vi "Simulation.Main.vi"() -> ()   [LabVIEW 2016, in "Simulation.lvclass"]
uses:
  Simulation.lvclass
  SimState.ctl
  Package ResourceControl/ViHandler/ViHandler.ViInfo.ctl
  SimModes.ctl
  Package Libraries/Message Queue/private/MessageQueue.MessageTypeDef.ctl
  <vilib>/Platform/TimedLoop/XDataNode/timing_clust.ctl
  <vilib>/Platform/TimedLoop/XDataNode/nitl_modes.ctl
  <vilib>/Platform/TimedLoop/XDataNode/wakeup.ctl
  Simulation.lvclass/Simulation.ctl
  Package ErrorHandling/ErrorHandling.lvclass/ErrorHandling.ctl
  Modell/Sondenmodell/Sondenmodell.lvclass/Sondenmodell.ctl
  Modell/Hausmodell/Hausmodell.lvclass/Hausmodell.ctl
  Modell/Umgebung/Umgebung.lvclass/Umgebung.ctl
  Package ErrorHandling/ErrorHandling.checkForErrorAndHandle.vi
  Package ErrorHandling/ErrorHandling.GetErrorHandler.vi
  <vilib>/Utility/error.llb/Clear Errors.vi
  Package Libraries/StringFunctions/StringFunctions_ReplaceAllBlindSigns.vi
  <vilib>/dlg_ctls.llb/Space Constant.vi
  <vilib>/Utility/error.llb/Error Cluster From Error Code.vi
  Package Libraries/TimingFunctions/TimingFunctions_getUtcTimestamp.vi
  <vilib>/Utility/error.llb/Trim Whitespace.vi
  <vilib>/Utility/error.llb/Search and Replace Pattern.vi
  Package ErrorHandling/ErrorHandling.addLastErrorToFile.vi
  <vilib>/ErrorRing/Error Ring.xnode
  Package ErrorHandling/ErrorHandling.lvclass
  <vilib>/Platform/TimedLoop/XDataNode/XDataNode.xnode
  <vilib>/Platform/TimedLoop/XDataNode/XDNodeRunTimeDep.lvlib
  Package ResourceControl/ViHandler/ViHandler.lvclass
  Modell/Sondenmodell/Sondenmodell.lvclass
  Modell/Umgebung/Umgebung.lvclass
  Modell/Hausmodell/Hausmodell.lvclass
panel:
  in  "Relative Zeit":timestamp=timestamp(3625116099.829659 s since 1904-01-01) format="%<%H:%M\n%d/%m/%Y>T"
  in  "Kalender und Uhrzeit Startwert":timestamp=timestamp(3625116099.829659 s since 1904-01-01) format="%<%H:%M\n%d/%m/%Y>T"
  in  "Umgebung":enum32{"Umgebung"}(tab)
  in  "Aussentemperatur [°C] Manuell":dbl(slide)=20.0 caption="Aussentemperatur [°C]" min=-20.0 max=40.0 scale=-20.0..40.0 scale format="%#.0f"
  in  "Manuelle Eingabe On/Off":bool
  out "Solare Gewinne [W]":dbl format="%#.0f"
  out "Strahlungsleistung  Sonne [W]":dbl format="%#.0f"
  in  "Kalender und Uhrzeit":timestamp=timestamp(3597606016.6082277 s since 1904-01-01) format="%<%H:%M\n%d/%m/%Y>T"
  out "Aussentemperatur":waveform(dbl)[](graph)
  in  "Solare Gewinne [W] Manuell":dbl(slide) caption="Solare Gewinne [W]" min=0.0 max=1000.0 scale=0.0..1000.0 scale format="%#.0f"
  in  "SimMode":T1
  in  "StopSim":bool
  in  "SimulationsModis":T2(tab)
  in  "Erdtemperatur [°C] Gesamtmodell":dbl=10.0 caption="Erdtemperatur [°C]" format="%#.0f"
  in  "Rücklauftemperatur Solekreislauf [°C] Gesamtmodell":dbl caption="Rücklauftemperatur Solekreislauf [°C]" format="%#.0f"
  in  "Rücklauftemperatur Heizkreislauf [°C] Gesamtmodell":dbl=25.0 caption="Rücklauftemperatur Heizkreislauf [°C]" format="%#.0f"
  in  "Bodentemperatur [°C] Gesamtmodell":dbl=20.0 caption="Bodentemperatur [°C]" format="%#.0f"
  in  "Raumtemperatur [°C] Gesamtmodell":dbl=15.0 caption="Raumtemperatur [°C]" format="%#.0f"
  in  "Verdichter 1 Gesamtmodell":bool caption="Verdichter 1"
  in  "Verdichter 2 Gesamtmodell":bool caption="Verdichter 2"
  out "Gesamtmodell":waveform(dbl)[](graph)
  out "Vorlauftemperatur Heizkreislauf [°C] Gesamtmodell":dbl=25.0 caption="Vorlauftemperatur Heizkreislauf [°C]" format="%#.0f"
  out "Vorlauftemperatur Solekreislauf [°C] Gesamtmodell":dbl caption="Vorlauftemperatur Solekreislauf [°C]" format="%#.0f"
  out "Hausmodell":waveform(dbl)[](graph)
  in  "Rücklauftemperatur Heizkreislauf [°C]":dbl=20.0 format="%#.0f"
  in  "Vorlauftemperatur \nHeizkreislauf [°C] Hausmodell":dbl(slide)=21.0 caption="Vorlauftemperatur \nHeizkreislauf [°C]" min=-20.0 max=60.0 scale=-20.0..60.0 scale format="%#_3p"
  in  "Bodentemperatur [°C]":dbl=18.0 format="%#.0f"
  in  "Raumtemperatur [°C]":dbl=16.0 format="%#.0f"
  in  "Erdtemperatur [°C]":dbl=10.0 min=0.0 max=20.0 format="%#.0f"
  in  "Rücklauftemperatur Solekreislauf [°C]":dbl=10.0 format="%#.0f"
  in  "Vorlauftemperatur \nSolekreislauf [°C] Sondemodell":dbl(slide)=9.0 caption="Vorlauftemperatur \nSolekreislauf [°C]" min=-10.0 max=20.0 scale=-10.0..20.0 scale format="%#.0f"
  out "Sondenmodell":waveform(dbl)[](graph)
  out "Vorlauftemperatur\n Solekreislauf [°C] Wärmepumpenmodell":dbl caption="Vorlauftemperatur\nSolekreislauf [°C]" format="%#.0f"
  out "Vorlauftemperatur\n Heizkreislauf [°C] Wärmepumpenmodell":dbl=35.0 caption="Vorlauftemperatur\nHeizkreislauf [°C]" format="%#.0f"
  out "Kälteleistung [W]":dbl format="%#.0f"
  out "Heizleistung [W]":dbl format="%#.0f"
  in  "Rücklauftemperatur \nSolekreislauf [°C] Wärmepumpenmodell":dbl(slide)=5.0 caption="Rücklauftemperatur \nSolekreislauf [°C]" min=-10.0 max=20.0 scale=-10.0..20.0 scale format="%#.0f"
  in  "Rücklauftemperatur Heizkreislauf  [°C] Wärmepumpenmodell":dbl(slide)=20.0 caption="Rücklauftemperatur \nHeizkreislauf [°C]" min=-20.0 max=60.0 scale=-20.0..60.0 scale format="%#.0f"
  in  "Verdichter 2 Wärmepumpenmodell":bool caption="Verdichter 2"
  in  "Verdichter 1 Wärmepumpenmodell":bool caption="Verdichter 1"
  out "ViInfo":T3
  in  "SetInitials":bool
  in  "PauseSim":bool
  in  "StartSim":bool
  in  "SimState":T4
  in  "Speed Multipier":i64=100
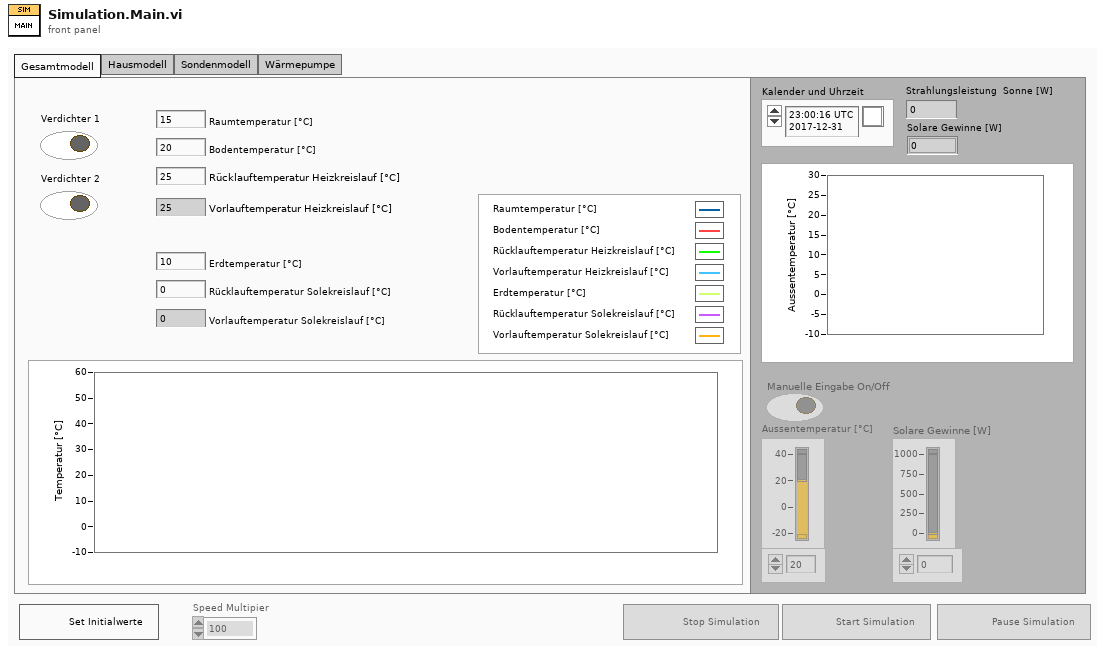
[diagram p1: front panel]
types:
  T1 = typedef "Simulation.lvclass/SimModes.ctl" = enum16{"Gesamtmodell", "HausOnly", "SondeOnly", "WPOnly"}
  T2 = enum32{"Gesamtmodell", "Hausmodell", "Sondenmodell", "Wärmepumpe"}
  T3 = typedef "ViHandler.lvclass/ViHandler.ViInfo.ctl" = cluster{"ViName":string, "ViReference":refnum<vi>, "ViQueueName":string}
  T4 = typedef "Simulation.lvclass/SimState.ctl" = enum16{"SetParams", "Running", "Idle", "Exit"}
  T5 = typedef "MessageQueue.MessageTypeDef.ctl" = cluster{"Message":string, "Data":variant}
  T6 = typedef "XDNodeRunTimeDep.lvlib/timing_clust.ctl" = cluster{"Expected End [f-1]":u64, "Actual End [f-1]":u64, "Finished Late? [f-1]":bool, "Expected End [i-1]":u64, "Actual End [i-1]":u64, "Finished Late? [i-1]":bool, "Expected Start [i]":u64, "Actual Start [i]":u64, "Expected Start [f]":u64, "Actual Start [f]":u64, "Source Name":string, "Structure Name":string, "Period":i64, "Deadline":i64, "Offset":i64, "Start":i64, "Priority":i32, "Timeout":i32, "Mode":T7, "Wakeup Reason":T8, "Error":errorcluster, "Source Type":string, "Secondary Source Type":string, "Global End Time":u64, "Global Start Time":u64, "Frame Duration":u64, "Iteration Duration":u64, "Assigned CPU":i32, "I/O Scan Engine Mode":u32}
  T7 = typedef "XDNodeRunTimeDep.lvlib/nitl_modes.ctl" = enum32{"No Change", "Process missed periods, maintain original phase", "Discard missed periods, maintain original phase", "Process missed periods, ignore original phase", "Discard missed periods, ignore original phase"}
  T8 = typedef "XDNodeRunTimeDep.lvlib/wakeup.ctl" = enum32{"Normal", "Aborted", "Asynchronous wakeup", "Timing source error", "Timed loop error", "Timeout"}
  T9 = enum8{"Enabled", "Disabled", "Disabled and Grayed Out"}
  T10 = enum32{"Page Enabled", "Page Disabled", "Page Disabled & Grayed"}
  T11 = typedef "Wärmepumpe.lvclass/Wärmepumpe.Zustandsgrössen.ctl" = cluster{"Vorlauftemperatur Heizkreislauf[°C]":dbl, "Vorlauftemperatur Solekreislauf[°C]":dbl, "Heizleistung [W]":dbl, "Kälteleistung [W]":dbl, "Verdichter 1":bool, "Verdichter 2":bool}
  T12 = typedef "Hausmodell.lvclass/Hausmodell.Zustandsgrössen.ctl" = cluster{"Raumtemperatur [°C]":dbl, "Bodentemperatur [°C]":dbl, "Rücklauftemperatur Heizkreislauf [°C]":dbl}
  T13 = typedef "Sondenmodell.lvclass/Sondenmodell.Zustandsgrössen.ctl" = cluster{"Erdtemperatur [°C]":dbl, "Rücklauftemperatur Solekreislauf [°C]":dbl}
  T14 = typedef "Umgebung.lvclass/Umgebung.Zustandsgrössen.ctl" = cluster{"Aussentemperatur [°C]":dbl, "Aussentemperatur [°C] Manuell":dbl, "Tag":dbl, "Stunde":dbl, "Minute":dbl, "Sekunden":dbl, "Strahlungsleistung [W]":dbl, "Solare Gewinne [W]":dbl, "Solare Gewinne [W] Manuell":dbl, "Manuelle Eingabe On/Off":bool}
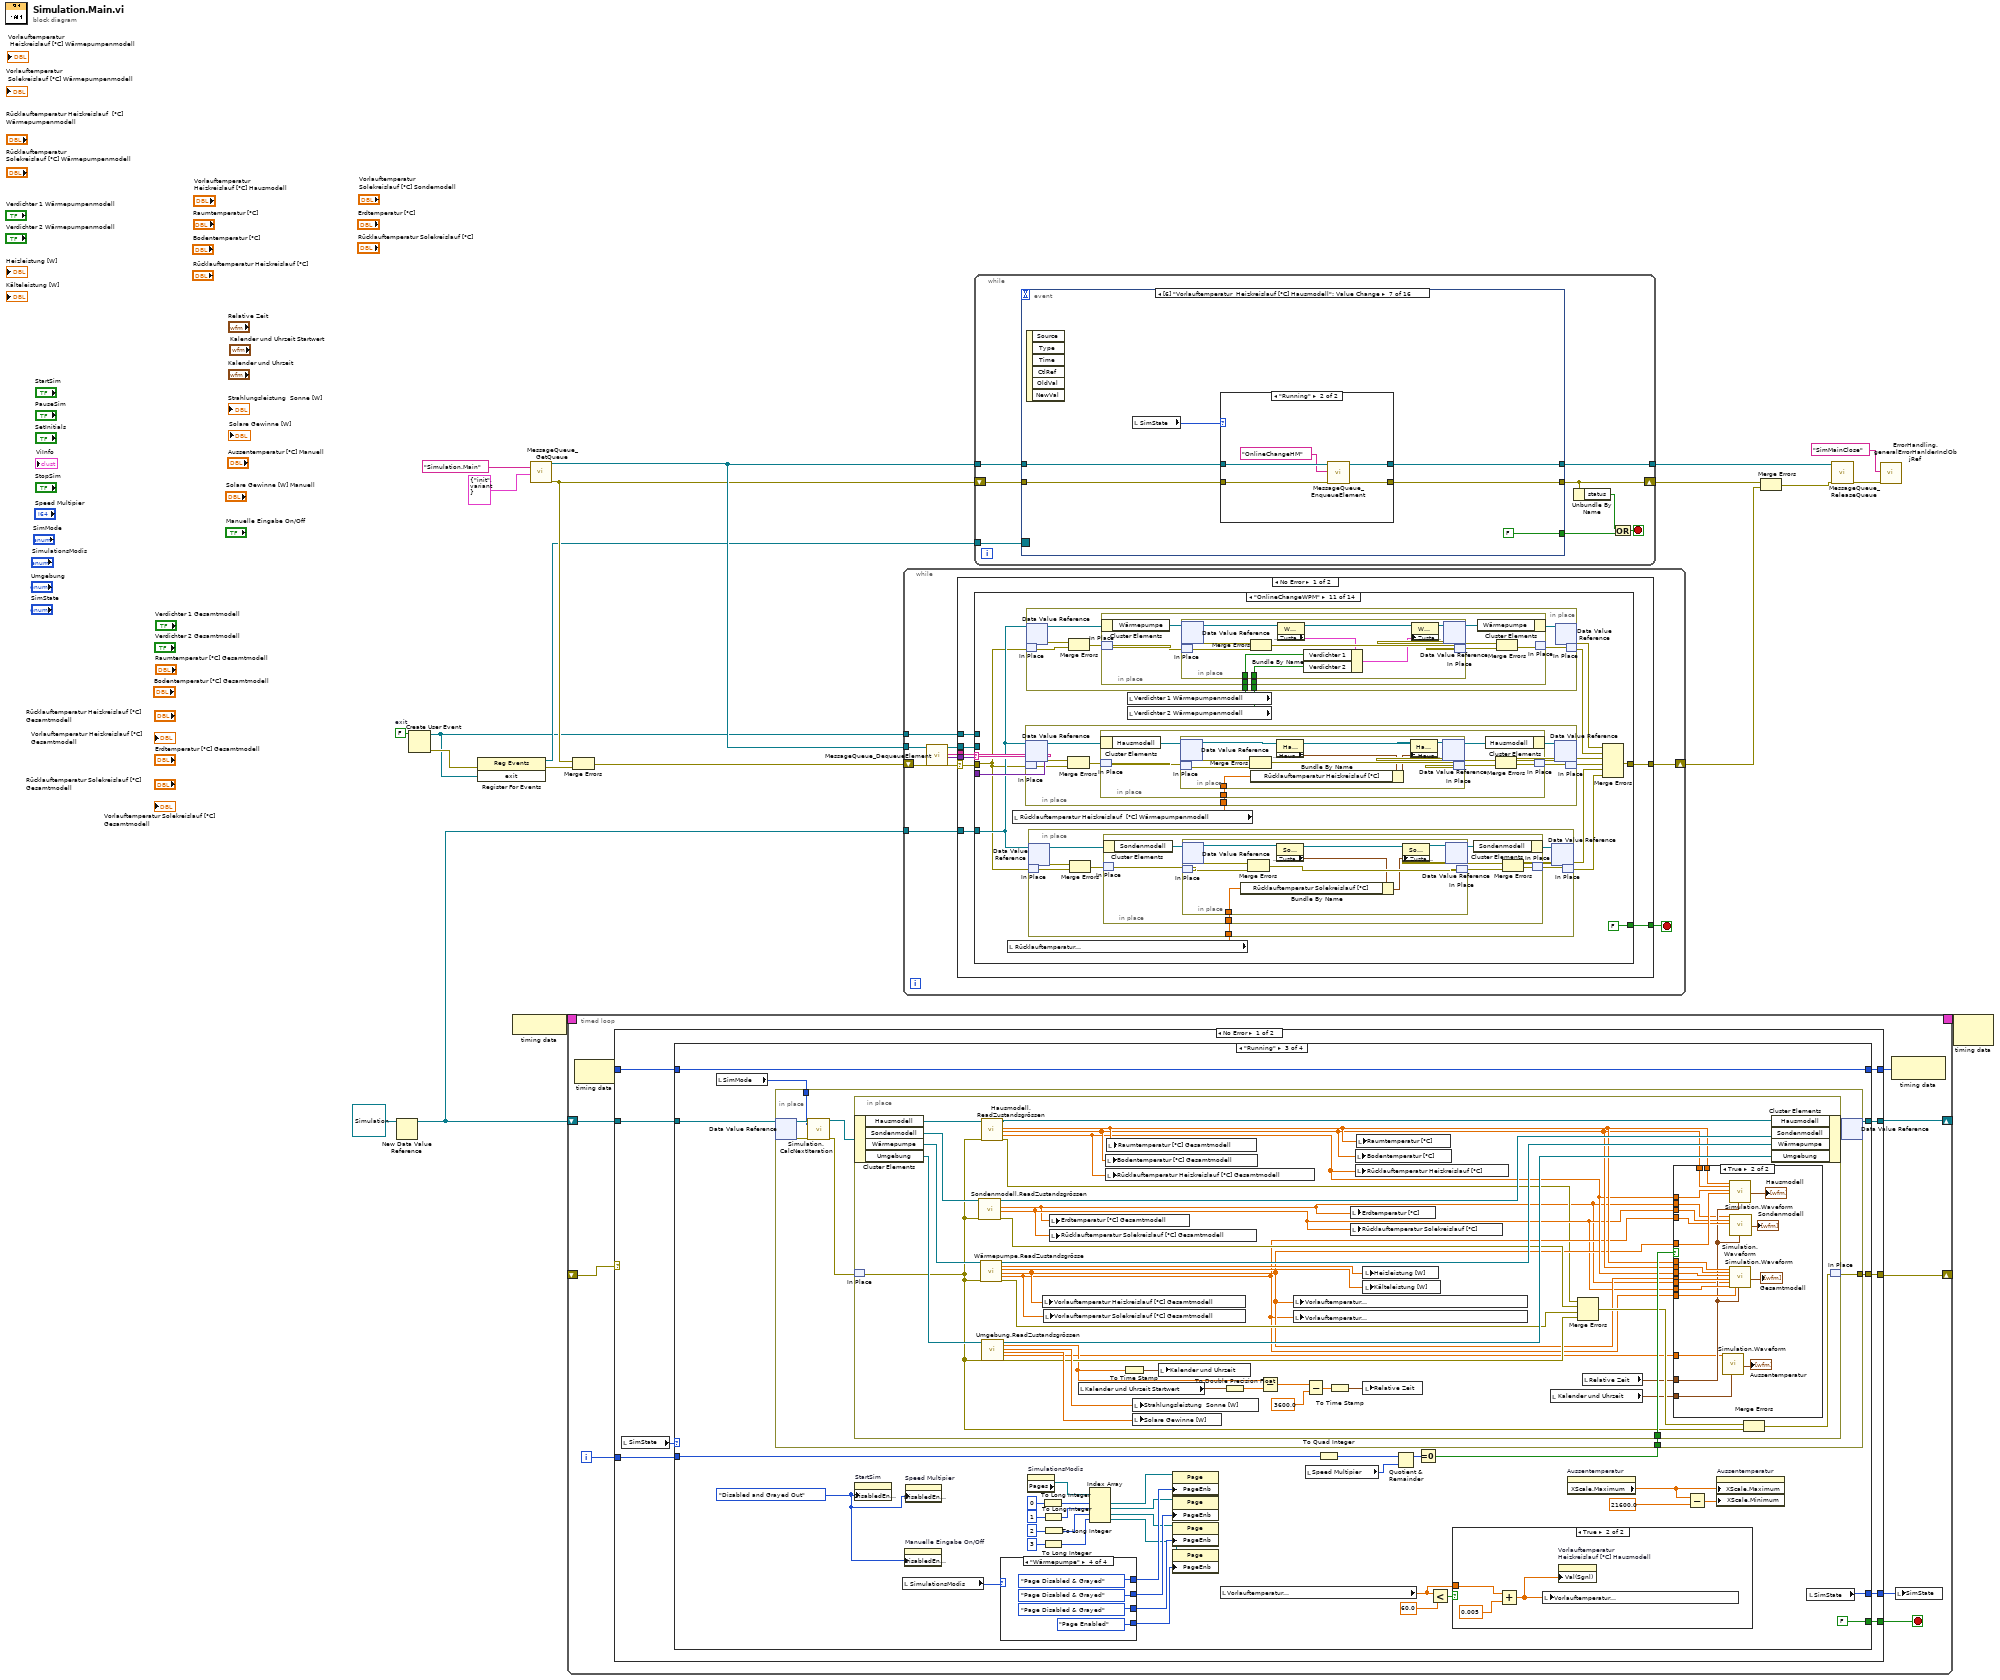
[diagram p0: block diagram]
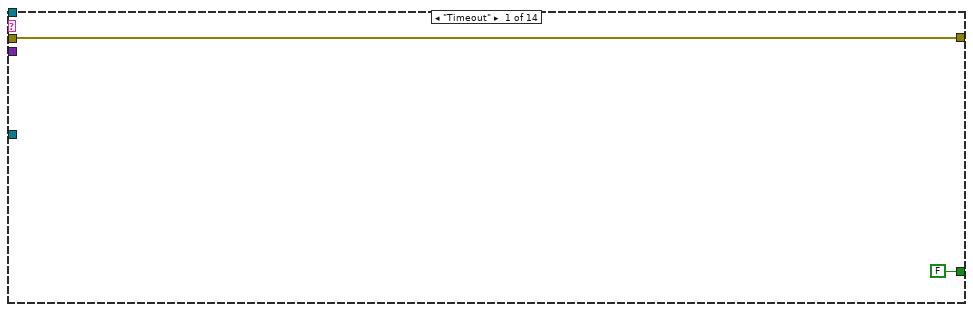
[diagram p2: hidden frame]
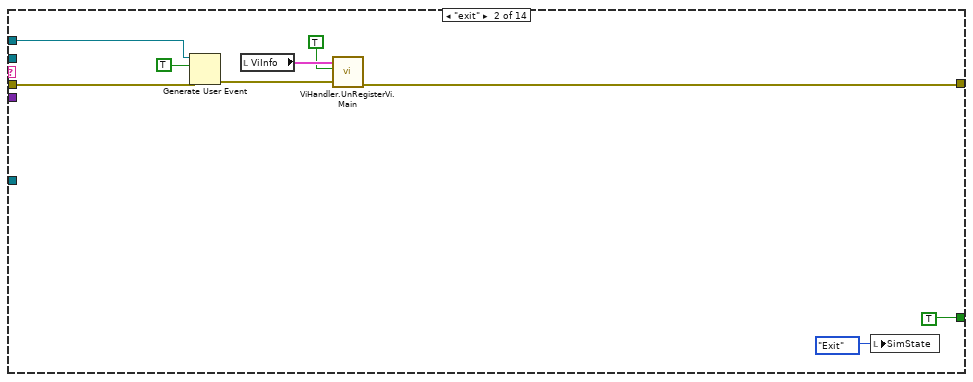
[diagram p3: hidden frame]
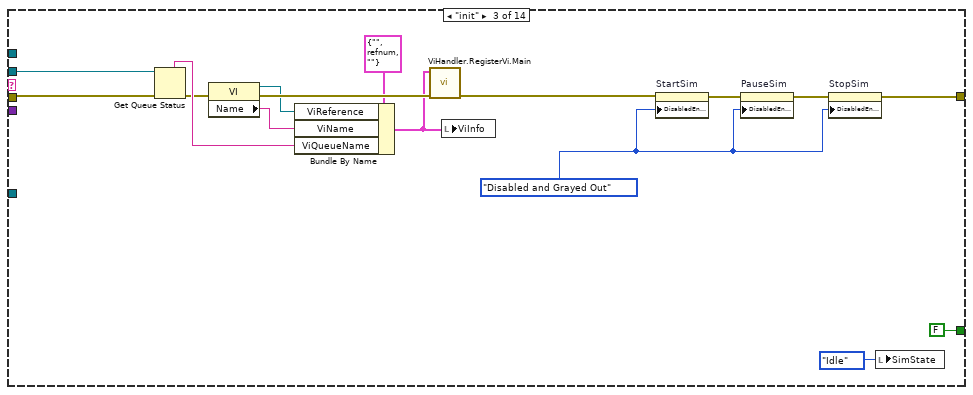
[diagram p4: hidden frame]
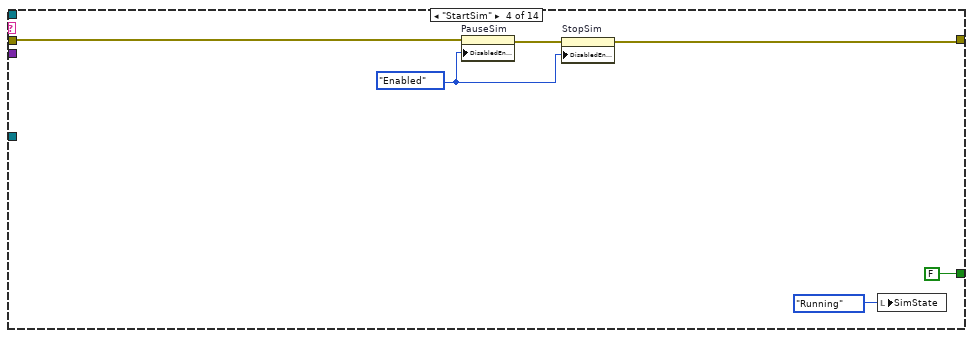
[diagram p5: hidden frame]
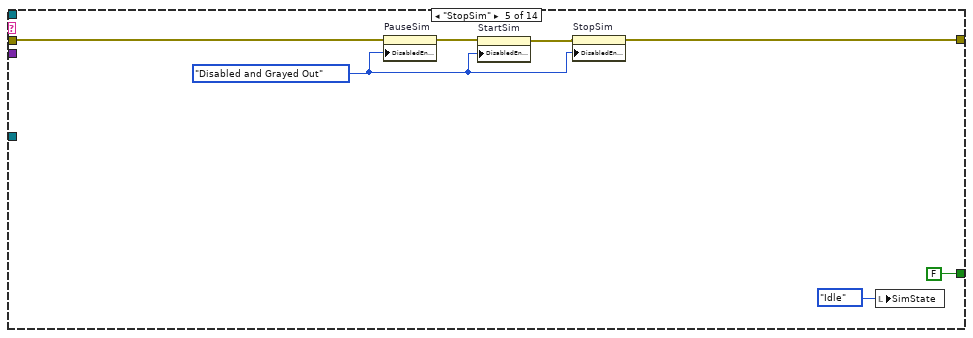
[diagram p6: hidden frame]
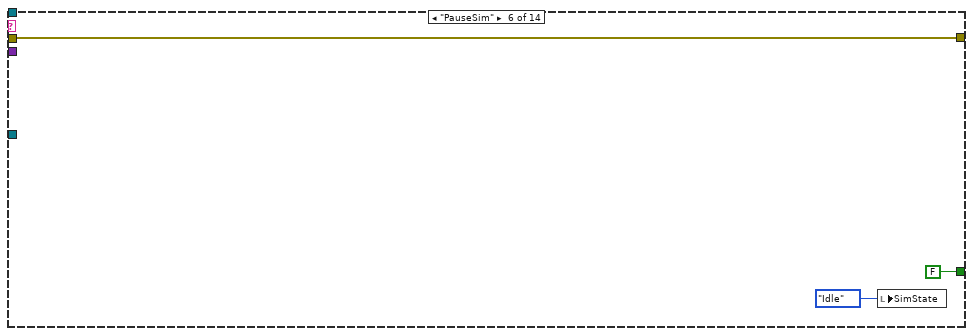
[diagram p7: hidden frame]
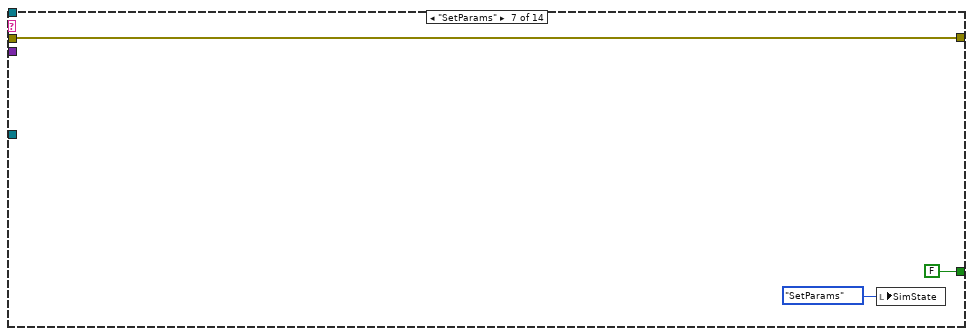
[diagram p8: hidden frame]
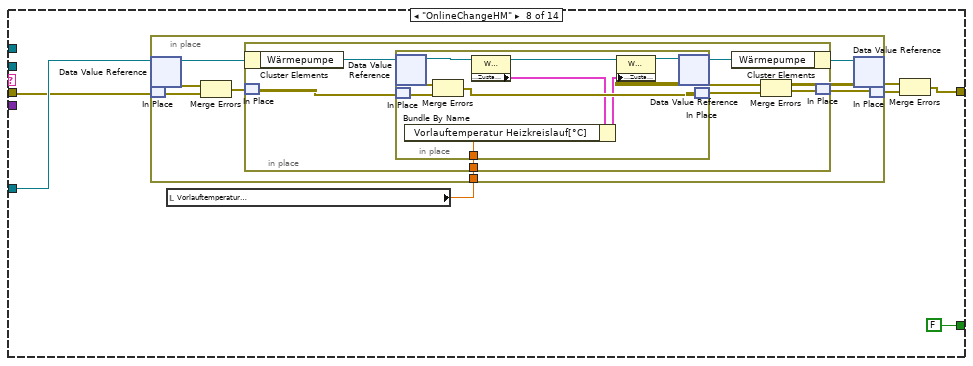
[diagram p9: hidden frame]
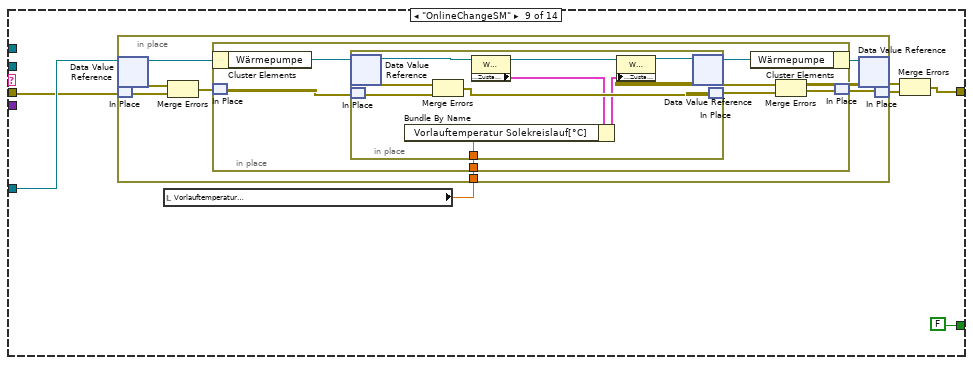
[diagram p10: hidden frame]
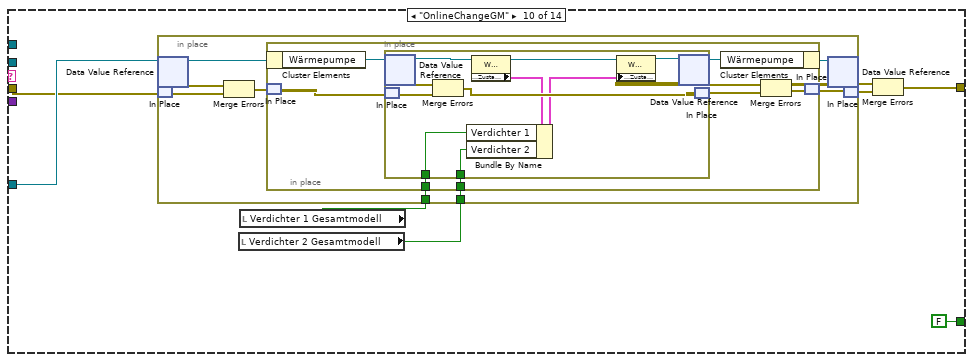
[diagram p11: hidden frame]
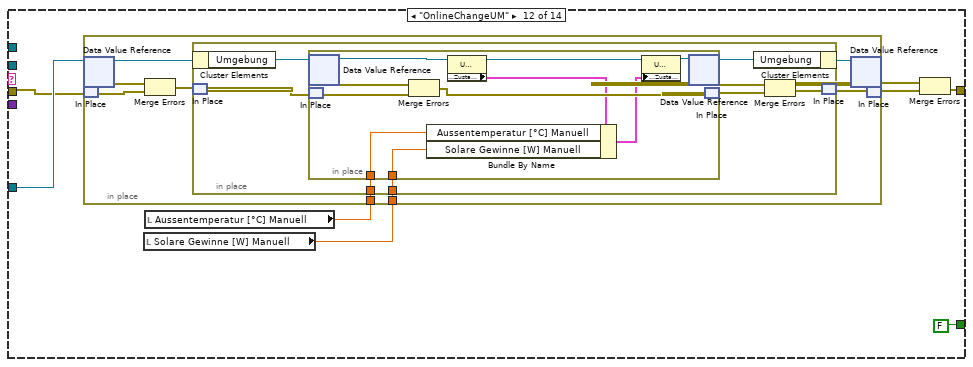
[diagram p12: hidden frame]
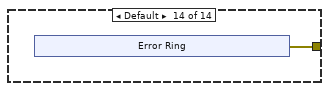
[diagram p14: hidden frame]
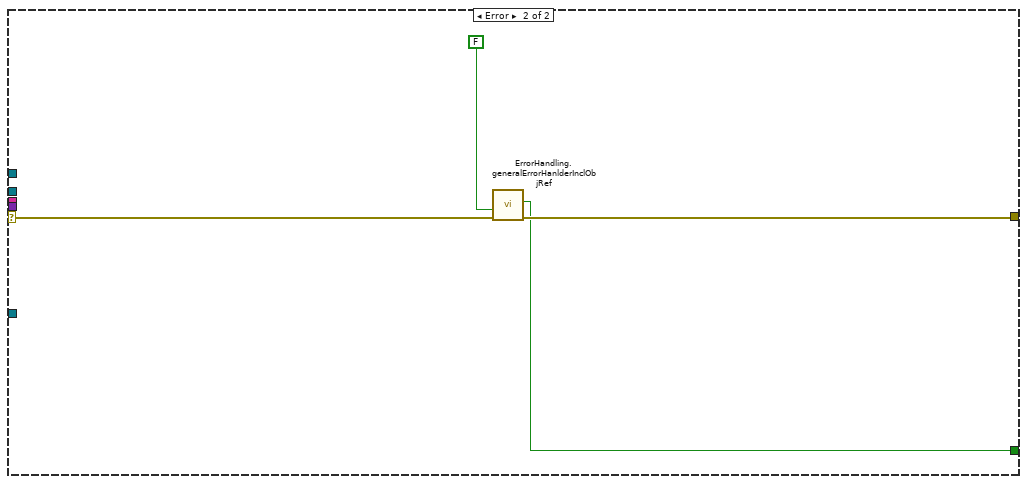
[diagram p15: hidden frame]
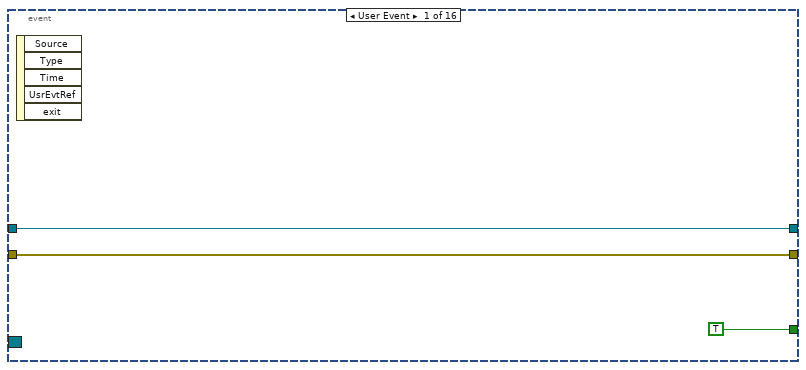
[diagram p16: hidden frame]
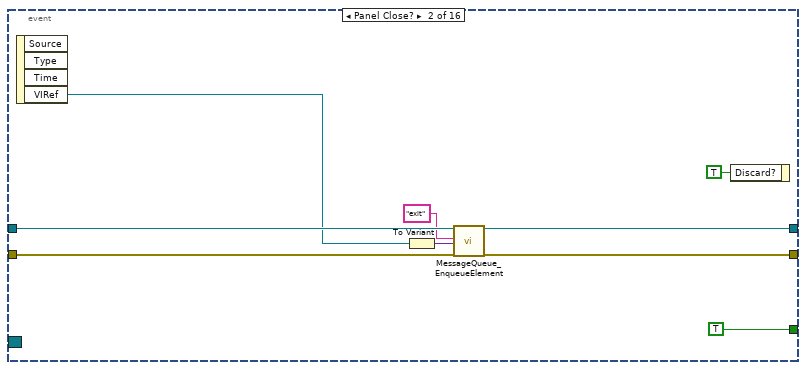
[diagram p17: hidden frame]
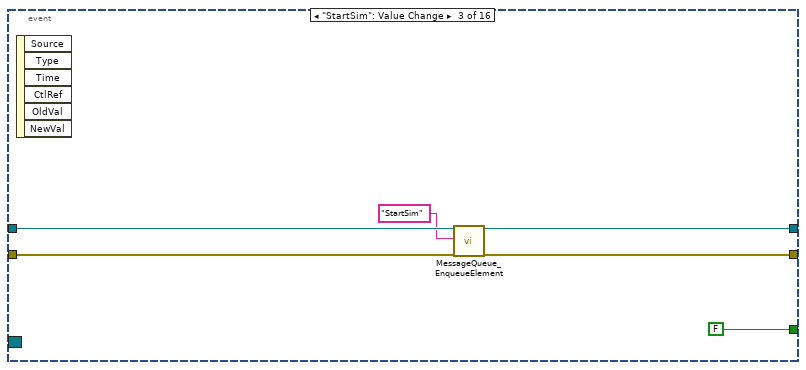
[diagram p18: hidden frame]
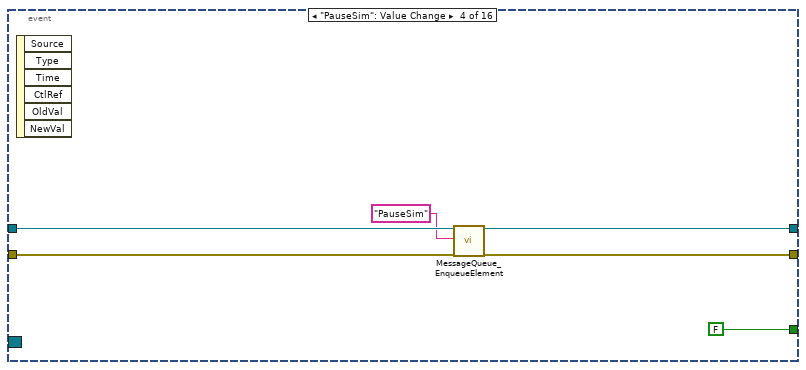
[diagram p19: hidden frame]
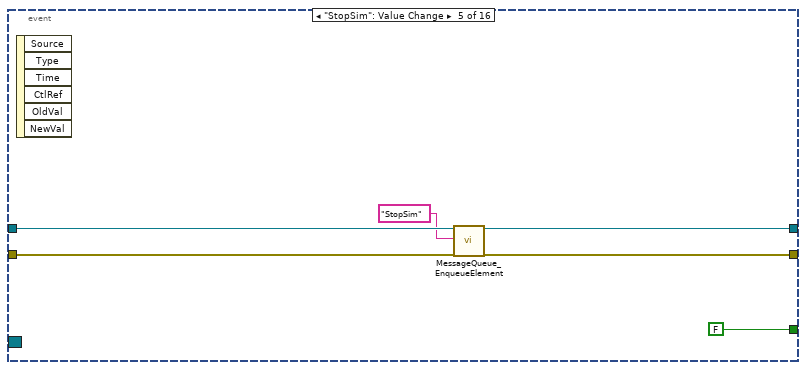
[diagram p20: hidden frame]
diagram:
  w13 = FALSE  # exit
  n1 = New Data Value Reference(data value=refnum<class "Simulation.lvclass"> refnum ("Simulation.lvclass")) -> (data value reference=w1:refnum<data-value>)  [unwired: 1 in, 1 out]
  n2 = Create User Event(user event datatype=w13) -> (user event=w11:refnum<user-event>, error out=w12:errorcluster)  [unwired: 1 in]
  n3 = register-events(error in=w12, w11) -> (reference out=w15:refnum<event-registration>, error out=w17:errorcluster)  [unwired: 1 in]
  n4 = node-c288() -> (w6:T6)
  n5 = call "MessageQueue_GetQueue.vi"("Name"="Simulation.Main", "OptionalInitValue"=T5 {"Message"="init", "Data"=variant}) -> ("QueueOut"=w19:refnum<queue>, "ErrorOut"=w16:errorcluster)  [unwired: 15 in, 1 out]
  n6 = timed-loop {
    timing: w6 -> [_]
    timing-out: [_] -> w5
    shift-right: [w28] -> _
    shift-left: w1 -> [w29]
    shift-right: [w23] -> _
    shift-left: _ -> [w22]
    i -> [w21]
    stop <- w26 stop-if-true
    n7 = node-c288() -> (w24:i64)  [unwired: 1 in]
    n8 = case shown="No Error" w22 {
      selector: w22 -> [_ w299]
      tunnel: w29 -> [w37 w298]
      tunnel: [w36 w298] -> w28
      tunnel: [w35 SimState."Idle" ("SimState")] -> w27
      tunnel: [w34 FALSE] -> w26
      tunnel: [w33 w295] -> w23
      tunnel: [w31 w297] -> w25
      tunnel: w24 -> [w32 w297]
      tunnel: w21 -> [w30 _]
      frame No Error {
        n9 = local read "SimState"() -> (w38:T4)
        n10 = case shown="\"Running\"" w38 {
          tunnel: w37 -> [w81 w160 w199 w293]
          tunnel: [w80 w160 w198 w293] -> w36
          tunnel: [SimState."Idle" ("SimState") w159 w201 SimState."Idle" ("SimState")] -> w35
          tunnel: [FALSE FALSE FALSE TRUE] -> w34
          tunnel: [w78 errorcluster {"status"=FALSE, "code"=0, "source"=""} ("error IO") w191 errorcluster {"status"=FALSE, "code"=0, "source"=""} ("error IO")] -> w33
          tunnel: [w65 w158 w197 w292] -> w31
          tunnel: w32 -> [_ w158 w197 w292]
          tunnel: w30 -> [_ _ w193 _]
          frame "SetParams" {
            n11 = local read "SimulationsModis"() -> (w50:T2)
            n12 = case shown="\"Gesamtmodell\", Default" w50 {
              tunnel: [SimModes."Gesamtmodell" ("SimMode") SimModes."HausOnly" ("SimMode") SimModes."SondeOnly" ("SimMode") SimModes."WPOnly" ("SimMode")] -> w51
              tunnel: [w92 w98 _ _] -> w49
              tunnel: [w91 w97 _ _] -> w48
              tunnel: [w87 w96 _ w110] -> w47
              tunnel: [w83 w94 _ w106] -> w46
              tunnel: [w90 _ w103 _] -> w45
              tunnel: [w85 _ w102 w109] -> w44
              tunnel: [w82 _ w100 w105] -> w43
              tunnel: [w89 _ _ w108] -> w42
              tunnel: [w88 _ _ w107] -> w41
              frame "Gesamtmodell", Default {
                n13 = local read "Raumtemperatur [°C] Gesamtmodell"() -> (w92:dbl)
                n14 = local read "Bodentemperatur [°C] Gesamtmodell"() -> (w91:dbl)
                n15 = local read "Rücklauftemperatur Heizkreislauf [°C] Gesamtmodell"() -> (w87:dbl)
                n16 = local read "Erdtemperatur [°C] Gesamtmodell"() -> (w90:dbl)
                n17 = local read "Rücklauftemperatur Solekreislauf [°C] Gesamtmodell"() -> (w85:dbl)
                n18 = local read "Verdichter 1 Gesamtmodell"() -> (w89:bool)
                n19 = local read "Verdichter 2 Gesamtmodell"() -> (w88:bool)
                n20 = Subtract(x=w85, y=1.0) -> (x-y=w82:dbl)
                n21 = local write "Vorlauftemperatur Solekreislauf [°C] Gesamtmodell"(w82) -> ()
                n22 = Add(x=w87, y=1.0) -> (x+y=w83:dbl)
                n23 = local write "Vorlauftemperatur Heizkreislauf [°C] Gesamtmodell"(w83) -> ()
              }
              frame "Hausmodell" {
                n24 = local read "Raumtemperatur [°C]"() -> (w98:dbl)
                n25 = local read "Bodentemperatur [°C]"() -> (w97:dbl)
                n26 = local read "Rücklauftemperatur Heizkreislauf [°C]"() -> (w96:dbl)
                n27 = Add(x=w96, y=1.0) -> (x+y=w94:dbl)
                n28 = local write "Vorlauftemperatur \nHeizkreislauf [°C] Hausmodell"(w94) -> ()
              }
              frame "Sondenmodell" {
                n29 = local read "Rücklauftemperatur Solekreislauf [°C]"() -> (w102:dbl)
                n30 = local read "Erdtemperatur [°C]"() -> (w103:dbl)
                n31 = Subtract(x=w102, y=1.0) -> (x-y=w100:dbl)
                n32 = local write "Vorlauftemperatur \nSolekreislauf [°C] Sondemodell"(w100) -> ()
              }
              frame "Wärmepumpe" {
                n33 = local read "Rücklauftemperatur \nSolekreislauf [°C] Wärmepumpenmodell"() -> (w109:dbl)
                n34 = local read "Rücklauftemperatur Heizkreislauf  [°C] Wärmepumpenmodell"() -> (w110:dbl)
                n35 = local read "Verdichter 1 Wärmepumpenmodell"() -> (w108:bool)
                n36 = local read "Verdichter 2 Wärmepumpenmodell"() -> (w107:bool)
                n37 = Subtract(x=w109, y=1.0) -> (x-y=w105:dbl)
                n38 = local write "Vorlauftemperatur\n Solekreislauf [°C] Wärmepumpenmodell"(w105) -> ()
                n39 = Add(x=w110, y=1.0) -> (x+y=w106:dbl)
                n40 = local write "Vorlauftemperatur\n Heizkreislauf [°C] Wärmepumpenmodell"(w106) -> ()
              }
            }
            n41 = local write "SimMode"(w51) -> ()
            n42 = local read "Solare Gewinne [W] Manuell"() -> (w56:dbl)
            n43 = local read "Aussentemperatur [°C] Manuell"() -> (w57:dbl)
            n44 = local read "Manuelle Eingabe On/Off"() -> (w40:bool)
            n45 = local read "Kalender und Uhrzeit"() -> (w39:timestamp)
            n46 = call "Hausmodell.GetRef.vi"() -> ("Error out"=w74:errorcluster, "Hausmodell"=w76:refnum<data-value>)  [unwired: 10 in]
            n47 = call "Sondenmodell.GetRef.vi"() -> ("Error out"=w61:errorcluster, "Sondenmodell"=w62:refnum<data-value>)  [unwired: 10 in]
            n48 = call "Wärmepumpe.GetRef.vi"() -> ("Error out"=w55:errorcluster, "Wärmepumpe"=w54:refnum<data-value>)  [unwired: 10 in]
            n49 = call "Umgebung.GetRef.vi"() -> ("Error out"=w69:errorcluster, "Umgebung"=w70:refnum<data-value>)  [unwired: 10 in]
            n50 = To Double Precision Float(number=w39) -> (double precision float=w63:dbl)
            n51 = call "Umgebung.WriteZustandsgrössen.vi"("Umgebung in"=w70, "Manuelle Eingabe On/Off"=w40, "Sekunden"=w63, "Aussentemperatur [°C] Manuell"=w57, "Solare Gewinne [W] Manuell"=w56, "Error in"=w69) -> ("Error out"=w59:errorcluster)  [unwired: 13 in]
            n52 = local write "Kalender und Uhrzeit Startwert"(w39) -> ()
            n53 = call "Hausmodell.WriteZustandsgrössen.vi"("Hausmodell in"=w76, "Raumtemperatur [°C]"=w49, "Bodentemperatur [°C]"=w48, "Rücklauftemperatur Heizkreislauf [°C]"=w47, "Error in"=w74) -> ("Error out"=w60:errorcluster)  [unwired: 14 in]
            n54 = call "Sondenmodell.WriteZustandsgrössen.vi"("Error in"=w61, "Rücklauftemperatur Solekreislauf [°C]"=w44, "Erdtemperatur [°C]"=w45, "Sondemodell in"=w62) -> ("Error out"=w52:errorcluster)  [unwired: 7 in]
            n55 = call "Wärmepumpe.WriteZustandsgrössen.vi"("Wärmepumpe in"=w54, "Vorlauftemperatur \nHeizkreislauf [°C] WPM"=w46, "Vorlauftemperatur \nSolekreislauf [°C] WPM"=w43, "Verdichter 1"=w42, "Verdichter 2"=w41, "Error in"=w55) -> ("Error out"=w53:errorcluster)  [unwired: 13 in]
            n56 = Merge Errors(w60, w52, w53, w59) -> (w58:errorcluster)
            n57 = in-place {
              n58 = in-place-dvr #1(w81) -> (w117:refnum<class "Simulation.lvclass">, w119:errorcluster)
              n59 = in-place-match #2(w58) -> (w118:errorcluster)
              n60 = Merge Errors(w119, w118) -> (w116:errorcluster)
              n61 = call "Simulation.SetAllObjectRefs.vi"("error in (no error)"=w116, "Simulation in"=w117) -> ("error out"=w115:errorcluster, "Simulation out"=w114:refnum<class "Simulation.lvclass">)  [unwired: 8 in]
              n62 = in-place-dvr #1(w114) -> (w80:refnum<data-value>, w79:errorcluster)
              n63 = in-place-match #2(w115) -> (w75:errorcluster)
            }
            n64 = property on="StartSim" class="Bool"("DisabledEnum"=T9."Enabled" ("Disabled")) -> (error out=w77:errorcluster)  [unwired: 2 in, 1 out]
            n65 = Merge Errors(w79, w75, w77) -> (w78:errorcluster)
            n66 = local read "Speed Multipier"() -> (w64:i64)
            n67 = To Double Precision Float(number=w64) -> (double precision float=w66:dbl)
            n68 = Divide(x=1000.0, y=w66) -> (x/y=w68:dbl)
            n69 = To Quad Integer(1:w68) -> (0:w65:i64)
          }
          frame "Idle", Default {
            w133 = T10."Page Enabled" ("Page Enabled State")
            w134 = T9."Enabled" ("Disabled")
            n70 = local read "Rücklauftemperatur Heizkreislauf  [°C] Wärmepumpenmodell"() -> (w139:dbl)
            n71 = local read "Rücklauftemperatur \nSolekreislauf [°C] Wärmepumpenmodell"() -> (w137:dbl)
            n72 = local read "Rücklauftemperatur Heizkreislauf [°C] Gesamtmodell"() -> (w152:dbl)
            n73 = local read "Rücklauftemperatur Solekreislauf [°C] Gesamtmodell"() -> (w150:dbl)
            n74 = local read "Rücklauftemperatur Heizkreislauf [°C]"() -> (w146:dbl)
            n75 = local read "Rücklauftemperatur Solekreislauf [°C]"() -> (w143:dbl)
            n76 = local read "Manuelle Eingabe On/Off"() -> (w155:bool)
            n77 = property on="Speed Multipier" class="DigNum (strict)"("DisabledEnum"=w134) -> ()  [unwired: 2 in, 2 out]
            n78 = property on="Manuelle Eingabe On/Off" class="Bool (strict)"("DisabledEnum"=w134) -> ()  [unwired: 2 in, 2 out]
            n79 = property on="SimulationsModis" class="TabCtl (strict)"("DisabledEnum"=w134) -> ()  [unwired: 2 in, 2 out]
            n80 = Add(x=w152, y=1.0) -> (x+y=w151:dbl)
            n81 = Subtract(x=w150, y=1.0) -> (x-y=w149:dbl)
            n82 = Add(x=w146, y=1.0) -> (x+y=w144:dbl)
            n83 = Subtract(x=w143, y=1.0) -> (x-y=w142:dbl)
            n84 = Add(x=w139, y=1.0) -> (x+y=w135:dbl)
            n85 = Subtract(x=w137, y=1.0) -> (x-y=w136:dbl)
            n86 = local write "Vorlauftemperatur Heizkreislauf [°C] Gesamtmodell"(w151) -> ()
            n87 = local write "Vorlauftemperatur Solekreislauf [°C] Gesamtmodell"(w149) -> ()
            n88 = local write "Vorlauftemperatur \nHeizkreislauf [°C] Hausmodell"(w144) -> ()
            n89 = local write "Vorlauftemperatur \nSolekreislauf [°C] Sondemodell"(w142) -> ()
            n90 = local write "Vorlauftemperatur\n Heizkreislauf [°C] Wärmepumpenmodell"(w135) -> ()
            n91 = local write "Vorlauftemperatur\n Solekreislauf [°C] Wärmepumpenmodell"(w136) -> ()
            n92 = case shown="False" w155 {
              tunnel: [T9."Disabled and Grayed Out" ("Disabled") T9."Enabled" ("Disabled")] -> w154
              tunnel: [T9."Enabled" ("Disabled") T9."Disabled and Grayed Out" ("Disabled")] -> w153
              frame False {
              }
              frame True {
              }
            }
            n93 = property on="Strahlungsleistung  Sonne [W]" class="DigNum (strict)"("DisabledEnum"=w153) -> ()  [unwired: 2 in, 2 out]
            n94 = property on="Solare Gewinne [W]" class="DigNum (strict)"("DisabledEnum"=w153) -> ()  [unwired: 2 in, 2 out]
            n95 = property on="Aussentemperatur [°C] Manuell" class="Slide (strict)"("DisabledEnum"=w154) -> ()  [unwired: 2 in, 2 out]
            n96 = property on="Solare Gewinne [W] Manuell" class="Slide (strict)"("DisabledEnum"=w154) -> ()  [unwired: 2 in, 2 out]
            n97 = property on="Kalender und Uhrzeit" class="AbsTime (strict)"("DisabledEnum"=w153) -> ()  [unwired: 2 in, 2 out]
            n98 = property on="Aussentemperatur" class="WFChart (strict)"("DisabledEnum"=w153) -> ()  [unwired: 2 in, 2 out]
            n99 = property on="SimulationsModis" class="TabCtl (strict)"() -> ("Pages"=w128:refnum<vi>[])  [unwired: 2 in, 2 out]
            n100 = To Long Integer(number=0) -> (32bit integer=w125:i32)
            n101 = To Long Integer(number=1) -> (32bit integer=w124:i32)
            n102 = To Long Integer(number=3) -> (32bit integer=w126:i32)
            n103 = To Long Integer(number=2) -> (32bit integer=w123:i32)
            n104 = Index Array(array=w128, index #1=w125, index #2=w124, index #3=w123, index #4=w126) -> (element #1=w129:refnum<vi>, element #2=w130:refnum<vi>, element #3=w131:refnum<vi>, element #4=w132:refnum<vi>)
            n105 = property class="Page"(reference=w129, "PageEnb"=w133) -> ()  [unwired: 1 in, 2 out]
            n106 = property class="Page"(reference=w130, "PageEnb"=w133) -> ()  [unwired: 1 in, 2 out]
            n107 = property class="Page"(reference=w131, "PageEnb"=w133) -> ()  [unwired: 1 in, 2 out]
            n108 = property class="Page"(reference=w132, "PageEnb"=w133) -> ()  [unwired: 1 in, 2 out]
            n109 = local read "SimState"() -> (w159:T4)
          }
          frame "Running" {
            w190 = T9."Disabled and Grayed Out" ("Disabled")
            n110 = local read "SimMode"() -> (w196:T1)
            n111 = property on="StartSim" class="Bool"("DisabledEnum"=w190) -> ()  [unwired: 2 in, 2 out]
            n112 = local read "SimulationsModis"() -> (w185:T2)
            n113 = property on="Manuelle Eingabe On/Off" class="Bool (strict)"("DisabledEnum"=w190) -> ()  [unwired: 2 in, 2 out]
            n114 = property on="Speed Multipier" class="DigNum (strict)"("DisabledEnum"=w190) -> ()  [unwired: 2 in, 2 out]
            n115 = case shown="\"Wärmepumpe\"" w185 {
              tunnel: [T10."Page Enabled" ("Page Enabled State") T10."Page Disabled & Grayed" ("Page Enabled State") T10."Page Disabled & Grayed" ("Page Enabled State") T10."Page Disabled & Grayed" ("Page Enabled State")] -> w186
              tunnel: [T10."Page Disabled & Grayed" ("Page Enabled State") T10."Page Enabled" ("Page Enabled State") T10."Page Disabled & Grayed" ("Page Enabled State") T10."Page Disabled & Grayed" ("Page Enabled State")] -> w187
              tunnel: [T10."Page Disabled & Grayed" ("Page Enabled State") T10."Page Disabled & Grayed" ("Page Enabled State") T10."Page Enabled" ("Page Enabled State") T10."Page Disabled & Grayed" ("Page Enabled State")] -> w188
              tunnel: [T10."Page Disabled & Grayed" ("Page Enabled State") T10."Page Disabled & Grayed" ("Page Enabled State") T10."Page Disabled & Grayed" ("Page Enabled State") T10."Page Enabled" ("Page Enabled State")] -> w189
              frame "Gesamtmodell", Default {
              }
              frame "Hausmodell" {
              }
              frame "Sondenmodell" {
              }
              frame "Wärmepumpe" {
              }
            }
            n116 = property on="SimulationsModis" class="TabCtl (strict)"() -> ("Pages"=w178:refnum<vi>[])  [unwired: 2 in, 2 out]
            n117 = To Long Integer(number=0) -> (32bit integer=w177:i32)
            n118 = To Long Integer(number=1) -> (32bit integer=w176:i32)
            n119 = To Long Integer(number=3) -> (32bit integer=w179:i32)
            n120 = To Long Integer(number=2) -> (32bit integer=w175:i32)
            n121 = Index Array(array=w178, index #1=w177, index #2=w176, index #3=w175, index #4=w179) -> (element #1=w181:refnum<vi>, element #2=w182:refnum<vi>, element #3=w183:refnum<vi>, element #4=w184:refnum<vi>)
            n122 = property class="Page"(reference=w181, "PageEnb"=w186) -> ()  [unwired: 1 in, 2 out]
            n123 = property class="Page"(reference=w182, "PageEnb"=w187) -> ()  [unwired: 1 in, 2 out]
            n124 = property class="Page"(reference=w183, "PageEnb"=w188) -> ()  [unwired: 1 in, 2 out]
            n125 = property class="Page"(reference=w184, "PageEnb"=w189) -> ()  [unwired: 1 in, 2 out]
            n126 = local read "Vorlauftemperatur \nHeizkreislauf [°C] Hausmodell"() -> (w170:dbl)
            n127 = local read "Speed Multipier"() -> (w171:i64)
            n128 = To Quad Integer(1:w193) -> (0:w194:i64)
            n129 = Quotient & Remainder(x=w194, y=w171) -> (x-y*floor(x/y)=w195:i64)  [unwired: 1 out]
            n130 = Equal To 0?(x=w195) -> (x = 0?=w192:bool)
            n131 = in-place {
              in-place-border: w196 -> [w221]
              in-place-border: [w223] -> w191
              in-place-border: w192 -> [w222]
              n132 = in-place-dvr #3(w199) -> (w227:refnum<class "Simulation.lvclass">, w225:errorcluster)
              n133 = call "Simulation.CalcNextIteration.vi"("Simulation in"=w227, "SimMode"=w221, "error in (no error)"=w225) -> ("Simulation out"=w226:refnum<class "Simulation.lvclass">, "error out"=w224:errorcluster)  [unwired: 15 in]
              n134 = in-place {
                in-place-border: w222 -> [w258]
                n135 = in-place-cluster #4(w226) -> ("Hausmodell"=w266:refnum<data-value>, "Sondenmodell"=w264:refnum<data-value>, "Wärmepumpe"=w262:refnum<data-value>, "Umgebung"=w260:refnum<data-value>)
                n136 = in-place-match #5(w224) -> (w250:errorcluster)
                n137 = call "Sondenmodell.ReadZustandsgrössen.vi"("Sondenmodell in"=w264, "error in"=w250) -> ("Sondenmodell out"=w263:refnum<data-value>, "Erdtemperatur [°C]"=w229:dbl, "Rücklauftemperatur Solekreislauf [°C]"=w231:dbl, "error out"=w252:errorcluster)  [unwired: 14 in]
                n138 = call "Wärmepumpe.ReadZustandsgrösse.vi"("Wärmepumpe in"=w262, "error in"=w250) -> ("Wärmepumpe out"=w261:refnum<data-value>, "Heizleistung [W]"=w248:dbl, "Kälteleistung [W]"=w257:dbl, "Vorlauftemperatur Heizkreislauf [°C]"=w235:dbl, "Vorlauftemperatur Solekreislauf [°C]"=w234:dbl, "error out"=w253:errorcluster)  [unwired: 10 in, 2 out]
                n139 = call "Hausmodell.ReadZustandsgrössen.vi"("Hausmodell in"=w266, "error in"=w250) -> ("Hausmodell out"=w265:refnum<data-value>, "Raumtemperatur [°C]"=w238:dbl, "Bodentemperatur [°C]"=w237:dbl, "Rücklauftemperatur Heizkreislauf [°C]"=w236:dbl, "error out"=w230:errorcluster)  [unwired: 13 in]
                n140 = call "Umgebung.ReadZustandsgrössen.vi"("Umgebung in"=w260, "error in"=w250) -> ("Umgebung out"=w259:refnum<data-value>, "Sekunden"=w239:dbl, "Strahlungsleistung [W]"=w255:dbl, "Solare Gewinne [W]"=w256:dbl, "Aussentemperatur [°C]"=w233:dbl, "error out"=w254:errorcluster)  [unwired: 12 in]
                n141 = local write "Vorlauftemperatur Heizkreislauf [°C] Gesamtmodell"(w235) -> ()
                n142 = local write "Vorlauftemperatur Solekreislauf [°C] Gesamtmodell"(w234) -> ()
                n143 = local write "Erdtemperatur [°C] Gesamtmodell"(w229) -> ()
                n144 = local write "Rücklauftemperatur Solekreislauf [°C] Gesamtmodell"(w231) -> ()
                n145 = local read "Kalender und Uhrzeit Startwert"() -> (w240:timestamp)
                n146 = local write "Bodentemperatur [°C] Gesamtmodell"(w237) -> ()
                n147 = local write "Rücklauftemperatur Heizkreislauf [°C] Gesamtmodell"(w236) -> ()
                n148 = local write "Raumtemperatur [°C] Gesamtmodell"(w238) -> ()
                n149 = To Time Stamp(1:w239) -> (0:w247:timestamp)
                n150 = local write "Strahlungsleistung  Sonne [W]"(w255) -> ()
                n151 = local write "Solare Gewinne [W]"(w256) -> ()
                n152 = local write "Kalender und Uhrzeit"(w247) -> ()
                n153 = To Double Precision Float(number=w240) -> (double precision float=w241:dbl)
                n154 = Subtract(x=w239, y=w241) -> (x-y=w244:dbl)
                n155 = local write "Vorlauftemperatur\n Heizkreislauf [°C] Wärmepumpenmodell"(w235) -> ()
                n156 = local write "Vorlauftemperatur\n Solekreislauf [°C] Wärmepumpenmodell"(w234) -> ()
                n157 = Subtract(x=w244, y=3600.0) -> (x-y=w243:dbl)
                n158 = To Time Stamp(1:w243) -> (0:w246:timestamp)
                n159 = local write "Erdtemperatur [°C]"(w229) -> ()
                n160 = local write "Rücklauftemperatur Solekreislauf [°C]"(w231) -> ()
                n161 = local write "Bodentemperatur [°C]"(w237) -> ()
                n162 = local write "Rücklauftemperatur Heizkreislauf [°C]"(w236) -> ()
                n163 = local write "Raumtemperatur [°C]"(w238) -> ()
                n164 = local write "Heizleistung [W]"(w248) -> ()
                n165 = local write "Kälteleistung [W]"(w257) -> ()
                n166 = local write "Relative Zeit"(w246) -> ()
                n167 = local read "Kalender und Uhrzeit"() -> (w232:timestamp)
                n168 = Merge Errors(w230, w252, w253, w254) -> (w251:errorcluster)
                n169 = local read "Relative Zeit"() -> (w245:timestamp)
                n170 = case shown="True" w258 {
                  tunnel: w233 -> [_ w267]
                  tunnel: w238 -> [_ w286]
                  tunnel: w237 -> [_ w285]
                  tunnel: w236 -> [_ w284]
                  tunnel: w235 -> [_ w283]
                  tunnel: w245 -> [_ w271]
                  tunnel: w231 -> [_ w281]
                  tunnel: w234 -> [_ w280]
                  tunnel: w238 -> [_ w278]
                  tunnel: w237 -> [_ w277]
                  tunnel: w236 -> [_ w276]
                  tunnel: w235 -> [_ w275]
                  tunnel: w231 -> [_ w274]
                  tunnel: w234 -> [_ w273]
                  tunnel: w232 -> [_ w268]
                  tunnel: w229 -> [_ w270]
                  tunnel: w229 -> [_ w269]
                  frame False {
                  }
                  frame True {
                    n171 = call "Simulation.Waveform.vi"("Temperatur 1 [°C]"=w267, "Zeit"=w268) -> ("Waveform Chart"=→"Aussentemperatur":waveform(dbl)[])  [unwired: 17 in]
                    n172 = call "Simulation.Waveform.vi"("Temperatur 1 [°C]"=w286, "Temperatur 2 [°C]"=w285, "Temperatur 3 [°C]"=w284, "Temperatur 4 [°C]"=w283, "Zeit"=w271) -> ("Waveform Chart"=→"Hausmodell":waveform(dbl)[])  [unwired: 14 in]
                    n173 = call "Simulation.Waveform.vi"("Temperatur 1 [°C]"=w278, "Temperatur 2 [°C]"=w277, "Temperatur 3 [°C]"=w276, "Temperatur 4 [°C]"=w275, "Temperatur 5 [°C]"=w269, "Temperatur 6 [°C]"=w274, "Temperatur 7 [°C]"=w273, "Zeit"=w271) -> ("Waveform Chart"=→"Gesamtmodell":waveform(dbl)[])  [unwired: 11 in]
                    n174 = call "Simulation.Waveform.vi"("Temperatur 1 [°C]"=w270, "Temperatur 2 [°C]"=w281, "Temperatur 3 [°C]"=w280, "Zeit"=w271) -> ("Waveform Chart"=→"Sondenmodell":waveform(dbl)[])  [unwired: 15 in]
                  }
                }
                n175 = Merge Errors(w251, w250) -> (w249:errorcluster)
                n176 = in-place-cluster #4("Hausmodell"=w265, "Sondenmodell"=w263, "Wärmepumpe"=w261, "Umgebung"=w259) -> (w228:refnum<class "Simulation.lvclass">)
                n177 = in-place-match #5(w249) -> (w223:errorcluster)
              }
              n178 = in-place-dvr #3(w228) -> (w198:refnum<data-value>)  [unwired: 1 out]
            }
            n179 = Less?(x=w170, y=60.0) -> (x < y?=w169:bool)
            n180 = case shown="True" w169 {
              tunnel: w170 -> [_ w203]
              frame False {
              }
              frame True {
                n181 = Add(x=w203, y=0.005) -> (x+y=w202:dbl)
                n182 = local write "Vorlauftemperatur \nHeizkreislauf [°C] Hausmodell"(w202) -> ()
                n183 = property on="Vorlauftemperatur \nHeizkreislauf [°C] Hausmodell" class="Slide (strict)"("Val(Sgnl)"=w202) -> ()  [unwired: 2 in, 2 out]
              }
            }
            n184 = property on="Aussentemperatur" class="WFChart (strict)"() -> ("XScale.Maximum"=w167:dbl)  [unwired: 2 in, 2 out]
            n185 = Subtract(x=w167, y=21600.0) -> (x-y=w166:dbl)
            n186 = property on="Aussentemperatur" class="WFChart (strict)"("XScale.Maximum"=w167, "XScale.Minimum"=w166) -> ()  [unwired: 2 in, 2 out]
            n187 = local read "SimState"() -> (w201:T4)
          }
          frame "Exit" {
            n188 = property on="SimulationsModis" class="TabCtl (strict)"("DisabledEnum"=T9."Enabled" ("Disabled")) -> ()  [unwired: 2 in, 2 out]
          }
        }
      }
      frame Error {
        n189 = call "ErrorHandling.generalErrorHanlderInclObjRef.vi"("error in"=w299) -> ("error out"=w295:errorcluster)  [unwired: 8 in, 2 out]
      }
    }
    n190 = node-c288(w25) -> ()  [unwired: 1 out]
    n191 = local write "SimState"(w27) -> ()
  }
  n192 = Merge Errors(w16, w17) -> (w14:errorcluster)
  n193 = while {
    tunnel: w19 -> [w314]
    tunnel: w11 -> [w307]
    shift-right: [w306] -> w9
    shift-left: w14 -> [w308]
    tunnel: w1 -> [w305]
    stop <- w309 stop-if-true
    n194 = call "MessageQueue_DequeueElement.vi"("QueueIn"=w314, "ErrorIn"=w308) -> ("QueueOut"=w312:refnum<queue>, "Message"=w311:string, "Data"=w310:variant, "ErrorOut"=w313:errorcluster)  [unwired: 13 in, 1 out]
    n195 = case shown="No Error" w313 {
      selector: w313 -> [w318 w593]
      tunnel: w312 -> [w322 _]
      tunnel: w311 -> [w321 _]
      tunnel: w310 -> [w320 _]
      tunnel: [w319 w591] -> w309
      tunnel: w307 -> [w317 _]
      tunnel: [w316 w592] -> w306
      tunnel: w305 -> [w315 _]
      frame No Error {
        n196 = case shown="\"OnlineChangeWPM\"" w321 {
          tunnel: w322 -> [_ _ w338 _ _ _ _ _ _ _ _ _ _ _]
          tunnel: w320 -> [_ _ _ _ _ _ _ _ _ _ _ _ _ _]
          tunnel: [FALSE TRUE FALSE FALSE FALSE FALSE FALSE FALSE FALSE FALSE FALSE FALSE _ _] -> w319
          tunnel: w318 -> [w323 w330 w340 w353 w360 w364 w367 w370 w400 w431 w467 w551 w583 _]
          tunnel: w317 -> [_ w326 _ _ _ _ _ _ _ _ _ _ _ _]
          tunnel: [w323 w328 w335 w350 w357 w364 w367 w371 w401 w432 w473 w553 w583 w584] -> w316
          tunnel: w315 -> [_ _ _ _ _ _ _ w374 w404 w435 w468 w552 _ _]
          frame "Timeout" {
          }
          frame "exit" {
            n197 = Generate User Event(user event=w326, event data cluster=TRUE ("event data"), error in=w330) -> (error out=w329:errorcluster)  [unwired: 1 in, 1 out]
            n198 = local read "ViInfo"() -> (w327:T3)
            n199 = call "ViHandler.UnRegisterVi.Main.vi"("ErrorIn"=w329, "FinalExit?"=TRUE, "ViInfo"=w327) -> ("ErrorOut"=w328:errorcluster)  [unwired: 7 in, 1 out]
            n200 = local write "SimState"(SimState."Exit" ("SimState")) -> ()
          }
          frame "init" {
            w334 = T9."Disabled and Grayed Out" ("Disabled")
            n201 = Get Queue Status(queue=w338, error in (no error)=w340) -> (queue name=w344:string, error out=w343:errorcluster)  [unwired: 1 in, 6 out]
            n202 = property class="VI"(error in=w343) -> (reference out=w342:refnum<vi>, error out=w346:errorcluster, "Name"=w341:string)  [unwired: 1 in]
            n203 = Bundle By Name(cluster=T3 {"ViName"="", "ViReference"=refnum, "ViQueueName"=""} ("ViInfo"), "ViReference"=w342, "ViName"=w341, "ViQueueName"=w344) -> (w337:T3)
            n204 = call "ViHandler.RegisterVi.Main.vi"("ErrorIn"=w346, "ViInfo"=w337) -> ("ErrorOut"=w339:errorcluster)  [unwired: 9 in]
            n205 = local write "ViInfo"(w337) -> ()
            n206 = property on="StartSim" class="Bool"(error in=w339, "DisabledEnum"=w334) -> (error out=w347:errorcluster)  [unwired: 1 in, 1 out]
            n207 = property on="PauseSim" class="Bool"(error in=w347, "DisabledEnum"=w334) -> (error out=w336:errorcluster)  [unwired: 1 in, 1 out]
            n208 = property on="StopSim" class="Bool"(error in=w336, "DisabledEnum"=w334) -> (error out=w335:errorcluster)  [unwired: 1 in, 1 out]
            n209 = local write "SimState"(SimState."Idle" ("SimState")) -> ()
          }
          frame "StartSim" {
            w352 = T9."Enabled" ("Disabled")
            n210 = property on="PauseSim" class="Bool"(error in=w353, "DisabledEnum"=w352) -> (error out=w351:errorcluster)  [unwired: 1 in, 1 out]
            n211 = property on="StopSim" class="Bool"(error in=w351, "DisabledEnum"=w352) -> (error out=w350:errorcluster)  [unwired: 1 in, 1 out]
            n212 = local write "SimState"(SimState."Running" ("SimState")) -> ()
          }
          frame "StopSim" {
            w356 = T9."Disabled and Grayed Out" ("Disabled")
            n213 = property on="PauseSim" class="Bool"(error in=w360, "DisabledEnum"=w356) -> (error out=w359:errorcluster)  [unwired: 1 in, 1 out]
            n214 = property on="StartSim" class="Bool"(error in=w359, "DisabledEnum"=w356) -> (error out=w358:errorcluster)  [unwired: 1 in, 1 out]
            n215 = property on="StopSim" class="Bool"(error in=w358, "DisabledEnum"=w356) -> (error out=w357:errorcluster)  [unwired: 1 in, 1 out]
            n216 = local write "SimState"(SimState."Idle" ("SimState")) -> ()
          }
          frame "PauseSim" {
            n217 = local write "SimState"(SimState."Idle" ("SimState")) -> ()
          }
          frame "SetParams" {
            n218 = local write "SimState"(SimState."SetParams" ("SimState")) -> ()
          }
          frame "OnlineChangeHM" {
            n219 = local read "Vorlauftemperatur \nHeizkreislauf [°C] Hausmodell"() -> (w369:dbl)
            n220 = in-place {
              in-place-border: w369 -> [w376]
              n221 = in-place-dvr #6(w374) -> (w380:refnum<class "Simulation.lvclass">, w382:errorcluster)
              n222 = in-place-match #7(w370) -> (w381:errorcluster)
              n223 = Merge Errors(w382, w381) -> (w378:errorcluster)
              n224 = in-place {
                in-place-border: w376 -> [w383]
                n225 = in-place-cluster #8(w380) -> ("Wärmepumpe"=w389:refnum<data-value>)
                n226 = in-place-match #9(w378) -> (w388:errorcluster)
                n227 = in-place {
                  in-place-border: w383 -> [w391]
                  n228 = in-place-dvr #10(w389) -> (w395:refnum<class "Wärmepumpe.lvclass">, w398:errorcluster)
                  n229 = in-place-match #11(w388) -> (w397:errorcluster)
                  n230 = Merge Errors(w398, w397) -> (w396:errorcluster)
                  n231 = property class="Wärmepumpe.lvclass"(reference=w395) -> (reference out=w394:refnum<class "Wärmepumpe.lvclass">, "Accessors:Wärmepumpe.Zustandsgrössen"=w390:T11)  [unwired: 1 in, 1 out]
                  n232 = Bundle By Name(cluster=w390, "Vorlauftemperatur Heizkreislauf[°C]"=w391) -> (w392:T11)
                  n233 = property class="Wärmepumpe.lvclass"(reference=w394, "Accessors:Wärmepumpe.Zustandsgrössen"=w392) -> (reference out=w393:refnum<class "Wärmepumpe.lvclass">)  [unwired: 1 in, 1 out]
                  n234 = in-place-dvr #10(w393) -> (w384:refnum<data-value>, w386:errorcluster)
                  n235 = in-place-match #11(w396) -> (w387:errorcluster)
                }
                n236 = in-place-cluster #8("Wärmepumpe"=w384) -> (w379:refnum<class "Simulation.lvclass">)
                n237 = Merge Errors(w386, w387) -> (w385:errorcluster)
                n238 = in-place-match #9(w385) -> (w377:errorcluster)
              }
              n239 = in-place-dvr #6(w379) -> (w373:errorcluster)  [unwired: 1 out]
              n240 = in-place-match #7(w377) -> (w372:errorcluster)
            }
            n241 = Merge Errors(w373, w372) -> (w371:errorcluster)
          }
          frame "OnlineChangeSM" {
            n242 = local read "Vorlauftemperatur \nSolekreislauf [°C] Sondemodell"() -> (w399:dbl)
            n243 = in-place {
              in-place-border: w399 -> [w406]
              n244 = in-place-dvr #12(w404) -> (w410:refnum<class "Simulation.lvclass">, w412:errorcluster)
              n245 = in-place-match #13(w400) -> (w411:errorcluster)
              n246 = Merge Errors(w412, w411) -> (w408:errorcluster)
              n247 = in-place {
                in-place-border: w406 -> [w413]
                n248 = in-place-cluster #14(w410) -> ("Wärmepumpe"=w419:refnum<data-value>)
                n249 = in-place-match #15(w408) -> (w418:errorcluster)
                n250 = in-place {
                  in-place-border: w413 -> [w421]
                  n251 = in-place-dvr #16(w419) -> (w425:refnum<class "Wärmepumpe.lvclass">, w428:errorcluster)
                  n252 = in-place-match #17(w418) -> (w427:errorcluster)
                  n253 = Merge Errors(w428, w427) -> (w426:errorcluster)
                  n254 = property class="Wärmepumpe.lvclass"(reference=w425) -> (reference out=w424:refnum<class "Wärmepumpe.lvclass">, "Accessors:Wärmepumpe.Zustandsgrössen"=w420:T11)  [unwired: 1 in, 1 out]
                  n255 = Bundle By Name(cluster=w420, "Vorlauftemperatur Solekreislauf[°C]"=w421) -> (w422:T11)
                  n256 = property class="Wärmepumpe.lvclass"(reference=w424, "Accessors:Wärmepumpe.Zustandsgrössen"=w422) -> (reference out=w423:refnum<class "Wärmepumpe.lvclass">)  [unwired: 1 in, 1 out]
                  n257 = in-place-dvr #16(w423) -> (w414:refnum<data-value>, w416:errorcluster)
                  n258 = in-place-match #17(w426) -> (w417:errorcluster)
                }
                n259 = in-place-cluster #14("Wärmepumpe"=w414) -> (w409:refnum<class "Simulation.lvclass">)
                n260 = Merge Errors(w416, w417) -> (w415:errorcluster)
                n261 = in-place-match #15(w415) -> (w407:errorcluster)
              }
              n262 = in-place-dvr #12(w409) -> (w403:errorcluster)  [unwired: 1 out]
              n263 = in-place-match #13(w407) -> (w402:errorcluster)
            }
            n264 = Merge Errors(w403, w402) -> (w401:errorcluster)
          }
          frame "OnlineChangeGM" {
            n265 = local read "Verdichter 2 Gesamtmodell"() -> (w430:bool)
            n266 = local read "Verdichter 1 Gesamtmodell"() -> (w429:bool)
            n267 = in-place {
              in-place-border: w430 -> [w438]
              in-place-border: w429 -> [w437]
              n268 = in-place-dvr #18(w435) -> (w442:refnum<class "Simulation.lvclass">, w444:errorcluster)
              n269 = in-place-match #19(w431) -> (w443:errorcluster)
              n270 = Merge Errors(w444, w443) -> (w440:errorcluster)
              n271 = in-place {
                in-place-border: w438 -> [w446]
                in-place-border: w437 -> [w445]
                n272 = in-place-cluster #20(w442) -> ("Wärmepumpe"=w452:refnum<data-value>)
                n273 = in-place-match #21(w440) -> (w451:errorcluster)
                n274 = in-place {
                  in-place-border: w446 -> [w454]
                  in-place-border: w445 -> [w453]
                  n275 = in-place-dvr #22(w452) -> (w459:refnum<class "Wärmepumpe.lvclass">, w462:errorcluster)
                  n276 = in-place-match #23(w451) -> (w461:errorcluster)
                  n277 = Merge Errors(w462, w461) -> (w460:errorcluster)
                  n278 = property class="Wärmepumpe.lvclass"(reference=w459) -> (reference out=w458:refnum<class "Wärmepumpe.lvclass">, "Accessors:Wärmepumpe.Zustandsgrössen"=w455:T11)  [unwired: 1 in, 1 out]
                  n279 = Bundle By Name(cluster=w455, "Verdichter 1"=w453, "Verdichter 2"=w454) -> (w456:T11)
                  n280 = property class="Wärmepumpe.lvclass"(reference=w458, "Accessors:Wärmepumpe.Zustandsgrössen"=w456) -> (reference out=w457:refnum<class "Wärmepumpe.lvclass">)  [unwired: 1 in, 1 out]
                  n281 = in-place-dvr #22(w457) -> (w447:refnum<data-value>, w449:errorcluster)
                  n282 = in-place-match #23(w460) -> (w450:errorcluster)
                }
                n283 = in-place-cluster #20("Wärmepumpe"=w447) -> (w441:refnum<class "Simulation.lvclass">)
                n284 = Merge Errors(w449, w450) -> (w448:errorcluster)
                n285 = in-place-match #21(w448) -> (w439:errorcluster)
              }
              n286 = in-place-dvr #18(w441) -> (w434:errorcluster)  [unwired: 1 out]
              n287 = in-place-match #19(w439) -> (w433:errorcluster)
            }
            n288 = Merge Errors(w434, w433) -> (w432:errorcluster)
          }
          frame "OnlineChangeWPM" {
            n289 = local read "Rücklauftemperatur \nSolekreislauf [°C] Wärmepumpenmodell"() -> (w470:dbl)
            n290 = local read "Rücklauftemperatur Heizkreislauf  [°C] Wärmepumpenmodell"() -> (w469:dbl)
            n291 = in-place {
              in-place-border: w469 -> [w503]
              n292 = in-place-dvr #24(w468) -> (w507:refnum<class "Simulation.lvclass">, w509:errorcluster)
              n293 = in-place-match #25(w467) -> (w508:errorcluster)
              n294 = Merge Errors(w509, w508) -> (w505:errorcluster)
              n295 = in-place {
                in-place-border: w503 -> [w510]
                n296 = in-place-cluster #26(w507) -> ("Hausmodell"=w516:refnum<data-value>)
                n297 = in-place-match #27(w505) -> (w515:errorcluster)
                n298 = in-place {
                  in-place-border: w510 -> [w519]
                  n299 = in-place-dvr #28(w516) -> (w522:refnum<class "Hausmodell.lvclass">, w525:errorcluster)
                  n300 = in-place-match #29(w515) -> (w524:errorcluster)
                  n301 = Merge Errors(w525, w524) -> (w523:errorcluster)
                  n302 = property class="Hausmodell.lvclass"(reference=w522) -> (reference out=w521:refnum<class "Hausmodell.lvclass">, "Accessors:Zustandsgrössen.Hausmodell"=w518:T12)  [unwired: 1 in, 1 out]
                  n303 = Bundle By Name(cluster=w518, "Rücklauftemperatur Heizkreislauf [°C]"=w519) -> (w517:T12)
                  n304 = property class="Hausmodell.lvclass"(reference=w521, "Accessors:Zustandsgrössen.Hausmodell"=w517) -> (reference out=w520:refnum<class "Hausmodell.lvclass">)  [unwired: 1 in, 1 out]
                  n305 = in-place-dvr #28(w520) -> (w511:refnum<data-value>, w513:errorcluster)
                  n306 = in-place-match #29(w523) -> (w514:errorcluster)
                }
                n307 = in-place-cluster #26("Hausmodell"=w511) -> (w506:refnum<class "Simulation.lvclass">)
                n308 = Merge Errors(w513, w514) -> (w512:errorcluster)
                n309 = in-place-match #27(w512) -> (w504:errorcluster)
              }
              n310 = in-place-dvr #24(w506) -> (w475:errorcluster)  [unwired: 1 out]
              n311 = in-place-match #25(w504) -> (w474:errorcluster)
            }
            n312 = in-place {
              in-place-border: w470 -> [w526]
              n313 = in-place-dvr #30(w468) -> (w530:refnum<class "Simulation.lvclass">, w532:errorcluster)
              n314 = in-place-match #31(w467) -> (w531:errorcluster)
              n315 = Merge Errors(w532, w531) -> (w528:errorcluster)
              n316 = in-place {
                in-place-border: w526 -> [w533]
                n317 = in-place-cluster #32(w530) -> ("Sondenmodell"=w539:refnum<data-value>)
                n318 = in-place-match #33(w528) -> (w538:errorcluster)
                n319 = in-place {
                  in-place-border: w533 -> [w540]
                  n320 = in-place-dvr #34(w539) -> (w545:refnum<class "Sondenmodell.lvclass">, w548:errorcluster)
                  n321 = in-place-match #35(w538) -> (w547:errorcluster)
                  n322 = Merge Errors(w548, w547) -> (w546:errorcluster)
                  n323 = property class="Sondenmodell.lvclass"(reference=w545) -> (reference out=w544:refnum<class "Sondenmodell.lvclass">, "Accessors:Sondenmodell.Zustandsgrössen"=w542:T13)  [unwired: 1 in, 1 out]
                  n324 = Bundle By Name(cluster=w542, "Rücklauftemperatur Solekreislauf [°C]"=w540) -> (w541:T13)
                  n325 = property class="Sondenmodell.lvclass"(reference=w544, "Accessors:Sondenmodell.Zustandsgrössen"=w541) -> (reference out=w543:refnum<class "Sondenmodell.lvclass">)  [unwired: 1 in, 1 out]
                  n326 = in-place-dvr #34(w543) -> (w534:refnum<data-value>, w536:errorcluster)
                  n327 = in-place-match #35(w546) -> (w537:errorcluster)
                }
                n328 = in-place-cluster #32("Sondenmodell"=w534) -> (w529:refnum<class "Simulation.lvclass">)
                n329 = Merge Errors(w536, w537) -> (w535:errorcluster)
                n330 = in-place-match #33(w535) -> (w527:errorcluster)
              }
              n331 = in-place-dvr #30(w529) -> (w472:errorcluster)  [unwired: 1 out]
              n332 = in-place-match #31(w527) -> (w471:errorcluster)
            }
            n333 = local read "Verdichter 1 Wärmepumpenmodell"() -> (w466:bool)
            n334 = local read "Verdichter 2 Wärmepumpenmodell"() -> (w465:bool)
            n335 = in-place {
              in-place-border: w466 -> [w478]
              in-place-border: w465 -> [w477]
              n336 = in-place-dvr #36(w468) -> (w482:refnum<class "Simulation.lvclass">, w484:errorcluster)
              n337 = in-place-match #37(w467) -> (w483:errorcluster)
              n338 = Merge Errors(w484, w483) -> (w480:errorcluster)
              n339 = in-place {
                in-place-border: w478 -> [w486]
                in-place-border: w477 -> [w485]
                n340 = in-place-cluster #38(w482) -> ("Wärmepumpe"=w492:refnum<data-value>)
                n341 = in-place-match #39(w480) -> (w491:errorcluster)
                n342 = in-place {
                  in-place-border: w486 -> [w494]
                  in-place-border: w485 -> [w493]
                  n343 = in-place-dvr #40(w492) -> (w499:refnum<class "Wärmepumpe.lvclass">, w502:errorcluster)
                  n344 = in-place-match #41(w491) -> (w501:errorcluster)
                  n345 = Merge Errors(w502, w501) -> (w500:errorcluster)
                  n346 = property class="Wärmepumpe.lvclass"(reference=w499) -> (reference out=w498:refnum<class "Wärmepumpe.lvclass">, "Accessors:Wärmepumpe.Zustandsgrössen"=w496:T11)  [unwired: 1 in, 1 out]
                  n347 = Bundle By Name(cluster=w496, "Verdichter 1"=w494, "Verdichter 2"=w493) -> (w495:T11)
                  n348 = property class="Wärmepumpe.lvclass"(reference=w498, "Accessors:Wärmepumpe.Zustandsgrössen"=w495) -> (reference out=w497:refnum<class "Wärmepumpe.lvclass">)  [unwired: 1 in, 1 out]
                  n349 = in-place-dvr #40(w497) -> (w487:refnum<data-value>, w489:errorcluster)
                  n350 = in-place-match #41(w500) -> (w490:errorcluster)
                }
                n351 = in-place-cluster #38("Wärmepumpe"=w487) -> (w481:refnum<class "Simulation.lvclass">)
                n352 = Merge Errors(w489, w490) -> (w488:errorcluster)
                n353 = in-place-match #39(w488) -> (w479:errorcluster)
              }
              n354 = in-place-dvr #36(w481) -> (w463:errorcluster)  [unwired: 1 out]
              n355 = in-place-match #37(w479) -> (w464:errorcluster)
            }
            n356 = Merge Errors(w463, w464, w475, w474, w472, w471) -> (w473:errorcluster)
          }
          frame "OnlineChangeUM" {
            n357 = local read "Solare Gewinne [W] Manuell"() -> (w549:dbl)
            n358 = local read "Aussentemperatur [°C] Manuell"() -> (w550:dbl)
            n359 = in-place {
              in-place-border: w550 -> [w558]
              in-place-border: w549 -> [w557]
              n360 = in-place-dvr #42(w552) -> (w562:refnum<class "Simulation.lvclass">, w564:errorcluster)
              n361 = in-place-match #43(w551) -> (w563:errorcluster)
              n362 = Merge Errors(w564, w563) -> (w560:errorcluster)
              n363 = in-place {
                in-place-border: w558 -> [w566]
                in-place-border: w557 -> [w565]
                n364 = in-place-cluster #44(w562) -> ("Umgebung"=w572:refnum<data-value>)
                n365 = in-place-match #45(w560) -> (w571:errorcluster)
                n366 = in-place {
                  in-place-border: w566 -> [w576]
                  in-place-border: w565 -> [w573]
                  n367 = in-place-dvr #46(w572) -> (w579:refnum<class "Umgebung.lvclass">, w582:errorcluster)
                  n368 = in-place-match #47(w571) -> (w581:errorcluster)
                  n369 = Merge Errors(w582, w581) -> (w580:errorcluster)
                  n370 = property class="Umgebung.lvclass"(reference=w579) -> (reference out=w578:refnum<class "Umgebung.lvclass">, "Accessors:Umgebung.Zustandsgrössen"=w575:T14)  [unwired: 1 in, 1 out]
                  n371 = Bundle By Name(cluster=w575, "Aussentemperatur [°C] Manuell"=w576, "Solare Gewinne [W] Manuell"=w573) -> (w574:T14)
                  n372 = property class="Umgebung.lvclass"(reference=w578, "Accessors:Umgebung.Zustandsgrössen"=w574) -> (reference out=w577:refnum<class "Umgebung.lvclass">)  [unwired: 1 in, 1 out]
                  n373 = in-place-dvr #46(w577) -> (w567:refnum<data-value>, w569:errorcluster)
                  n374 = in-place-match #47(w580) -> (w570:errorcluster)
                }
                n375 = in-place-cluster #44("Umgebung"=w567) -> (w561:refnum<class "Simulation.lvclass">)
                n376 = Merge Errors(w569, w570) -> (w568:errorcluster)
                n377 = in-place-match #45(w568) -> (w559:errorcluster)
              }
              n378 = in-place-dvr #42(w561) -> (w555:errorcluster)  [unwired: 1 out]
              n379 = in-place-match #43(w559) -> (w554:errorcluster)
            }
            n380 = Merge Errors(w555, w554) -> (w553:errorcluster)
          }
          frame "UpdateGUI" {
          }
          frame Default {
            n381 = xnode "Error Ring"() -> ("error out"=w584:errorcluster)
          }
        }
      }
      frame Error {
        n382 = call "ErrorHandling.generalErrorHanlderInclObjRef.vi"("error in"=w593, "StopOnError"=FALSE) -> ("error out"=w592:errorcluster, "Stop"=w591:bool)  [unwired: 7 in, 1 out]
      }
    }
  }
  n383 = while {
    tunnel: w19 -> [w601]
    tunnel: [w600] -> w20
    shift-right: [w597] -> w8
    shift-left: w16 -> [w599]
    tunnel: w15 -> [w594]
    stop <- w596 stop-if-true
    n384 = event shown="[6] \"Vorlauftemperatur  Heizkreislauf [°C] Hausmodell\": Value Change" {
      selector: w594 -> [_ _ _ _ _ _ _ _ _ _ _ _ _ _ _ _]
      dyn-events: _ -> [_ _ _ _ _ _ _ _ _ _ _ _ _ _ _ _]
      timeout: _ -> [_ _ _ _ _ _ _ _ _ _ _ _ _ _ _ _]
      tunnel: w601 -> [w603 w613 w619 w625 w631 w637 w643 w656 w669 w682 w695 w708 w721 w734 w747 w760]
      tunnel: [w603 w612 w618 w624 w630 w636 w642 w655 w668 w681 w694 w707 w720 w733 w746 w759] -> w600
      tunnel: [w602 w605 w614 w620 w626 w632 w639 w652 w665 w678 w691 w704 w717 w730 w743 w756] -> w597
      tunnel: w599 -> [w602 w608 w615 w621 w627 w633 w640 w653 w666 w679 w692 w705 w718 w731 w744 w757]
      tunnel: [TRUE TRUE FALSE FALSE FALSE FALSE FALSE FALSE FALSE FALSE FALSE FALSE FALSE FALSE FALSE FALSE] -> w598
      event User Event {
        n385 = event-data() -> ()  [unwired: 1 in, 5 out]
      }
      event Panel Close? {
        n386 = event-data() -> ("VIRef"=w606:refnum<vi>)  [unwired: 1 in, 3 out]
        n387 = To Variant(anything=w606) -> (Variant=w607:variant)
        n388 = call "MessageQueue_EnqueueElement.vi"("QueueIn"=w613, "Message"="exit", "Data"=w607, "ErrorIn"=w608) -> ("QueueOut"=w612:refnum<queue>, "ErrorOut"=w605:errorcluster)  [unwired: 14 in]
        n389 = event-data("Discard?"=TRUE) -> ()  [unwired: 1 in, 1 out]
      }
      event "StartSim": Value Change {
        n390 = event-data() -> ()  [unwired: 1 in, 6 out]
        n391 = call "MessageQueue_EnqueueElement.vi"("QueueIn"=w619, "Message"="StartSim", "ErrorIn"=w615) -> ("QueueOut"=w618:refnum<queue>, "ErrorOut"=w614:errorcluster)  [unwired: 15 in]
      }
      event "PauseSim": Value Change {
        n392 = event-data() -> ()  [unwired: 1 in, 6 out]
        n393 = call "MessageQueue_EnqueueElement.vi"("QueueIn"=w625, "Message"="PauseSim", "ErrorIn"=w621) -> ("QueueOut"=w624:refnum<queue>, "ErrorOut"=w620:errorcluster)  [unwired: 15 in]
      }
      event "StopSim": Value Change {
        n394 = event-data() -> ()  [unwired: 1 in, 6 out]
        n395 = call "MessageQueue_EnqueueElement.vi"("QueueIn"=w631, "Message"="StopSim", "ErrorIn"=w627) -> ("QueueOut"=w630:refnum<queue>, "ErrorOut"=w626:errorcluster)  [unwired: 15 in]
      }
      event "SetInitials": Value Change {
        n396 = event-data() -> ()  [unwired: 1 in, 6 out]
        n397 = call "MessageQueue_EnqueueElement.vi"("QueueIn"=w637, "Message"="SetParams", "ErrorIn"=w633) -> ("QueueOut"=w636:refnum<queue>, "ErrorOut"=w632:errorcluster)  [unwired: 15 in]
      }
      event "Vorlauftemperatur \nHeizkreislauf [°C] Hausmodell": Value Change {
        n398 = event-data() -> ()  [unwired: 1 in, 6 out]
        n399 = local read "SimState"() -> (w638:T4)
        n400 = case shown="\"Running\"" w638 {
          tunnel: w643 -> [w645 w650]
          tunnel: [w645 w649] -> w642
          tunnel: w640 -> [w644 w647]
          tunnel: [w644 w646] -> w639
          frame Default {
          }
          frame "Running" {
            n401 = call "MessageQueue_EnqueueElement.vi"("QueueIn"=w650, "Message"="OnlineChangeHM", "ErrorIn"=w647) -> ("QueueOut"=w649:refnum<queue>, "ErrorOut"=w646:errorcluster)  [unwired: 15 in]
          }
        }
      }
      event "Vorlauftemperatur \nSolekreislauf [°C] Sondemodell": Value Change {
        n402 = event-data() -> ()  [unwired: 1 in, 6 out]
        n403 = local read "SimState"() -> (w651:T4)
        n404 = case shown="\"Running\"" w651 {
          tunnel: w656 -> [w658 w663]
          tunnel: [w658 w662] -> w655
          tunnel: w653 -> [w657 w660]
          tunnel: [w657 w659] -> w652
          frame Default {
          }
          frame "Running" {
            n405 = call "MessageQueue_EnqueueElement.vi"("QueueIn"=w663, "Message"="OnlineChangeSM", "ErrorIn"=w660) -> ("QueueOut"=w662:refnum<queue>, "ErrorOut"=w659:errorcluster)  [unwired: 15 in]
          }
        }
      }
      event "Rücklauftemperatur Heizkreislauf  [°C] Wärmepumpenmodell": Value Change {
        n406 = event-data() -> ()  [unwired: 1 in, 6 out]
        n407 = local read "SimState"() -> (w664:T4)
        n408 = case shown="\"Running\"" w664 {
          tunnel: w669 -> [w671 w676]
          tunnel: [w671 w675] -> w668
          tunnel: w666 -> [w670 w673]
          tunnel: [w670 w672] -> w665
          frame Default {
          }
          frame "Running" {
            n409 = call "MessageQueue_EnqueueElement.vi"("QueueIn"=w676, "Message"="OnlineChangeWPM", "ErrorIn"=w673) -> ("QueueOut"=w675:refnum<queue>, "ErrorOut"=w672:errorcluster)  [unwired: 15 in]
          }
        }
      }
      event "Rücklauftemperatur \nSolekreislauf [°C] Wärmepumpenmodell": Value Change {
        n410 = event-data() -> ()  [unwired: 1 in, 6 out]
        n411 = local read "SimState"() -> (w677:T4)
        n412 = case shown="\"Running\"" w677 {
          tunnel: w682 -> [w684 w689]
          tunnel: [w684 w688] -> w681
          tunnel: w679 -> [w683 w686]
          tunnel: [w683 w685] -> w678
          frame Default {
          }
          frame "Running" {
            n413 = call "MessageQueue_EnqueueElement.vi"("QueueIn"=w689, "Message"="OnlineChangeWPM", "ErrorIn"=w686) -> ("QueueOut"=w688:refnum<queue>, "ErrorOut"=w685:errorcluster)  [unwired: 15 in]
          }
        }
      }
      event "Verdichter 1 Wärmepumpenmodell": Value Change {
        n414 = event-data() -> ()  [unwired: 1 in, 6 out]
        n415 = local read "SimState"() -> (w690:T4)
        n416 = case shown="\"Running\"" w690 {
          tunnel: w695 -> [w697 w702]
          tunnel: [w697 w701] -> w694
          tunnel: w692 -> [w696 w699]
          tunnel: [w696 w698] -> w691
          frame Default {
          }
          frame "Running" {
            n417 = call "MessageQueue_EnqueueElement.vi"("QueueIn"=w702, "Message"="OnlineChangeWPM", "ErrorIn"=w699) -> ("QueueOut"=w701:refnum<queue>, "ErrorOut"=w698:errorcluster)  [unwired: 15 in]
          }
        }
      }
      event "Verdichter 2 Wärmepumpenmodell": Value Change {
        n418 = event-data() -> ()  [unwired: 1 in, 6 out]
        n419 = local read "SimState"() -> (w703:T4)
        n420 = case shown="\"Running\"" w703 {
          tunnel: w708 -> [w710 w715]
          tunnel: [w710 w714] -> w707
          tunnel: w705 -> [w709 w712]
          tunnel: [w709 w711] -> w704
          frame Default {
          }
          frame "Running" {
            n421 = call "MessageQueue_EnqueueElement.vi"("QueueIn"=w715, "Message"="OnlineChangeWPM", "ErrorIn"=w712) -> ("QueueOut"=w714:refnum<queue>, "ErrorOut"=w711:errorcluster)  [unwired: 15 in]
          }
        }
      }
      event "Aussentemperatur [°C] Manuell": Value Change {
        n422 = event-data() -> ()  [unwired: 1 in, 6 out]
        n423 = local read "SimState"() -> (w716:T4)
        n424 = case shown="\"Running\"" w716 {
          tunnel: w721 -> [w723 w728]
          tunnel: [w723 w727] -> w720
          tunnel: w718 -> [w722 w725]
          tunnel: [w722 w724] -> w717
          frame Default {
          }
          frame "Running" {
            n425 = call "MessageQueue_EnqueueElement.vi"("QueueIn"=w728, "Message"="OnlineChangeUM", "ErrorIn"=w725) -> ("QueueOut"=w727:refnum<queue>, "ErrorOut"=w724:errorcluster)  [unwired: 15 in]
          }
        }
      }
      event "Solare Gewinne [W] Manuell": Value Change {
        n426 = event-data() -> ()  [unwired: 1 in, 6 out]
        n427 = local read "SimState"() -> (w729:T4)
        n428 = case shown="\"Running\"" w729 {
          tunnel: w734 -> [w736 w741]
          tunnel: [w736 w740] -> w733
          tunnel: w731 -> [w735 w738]
          tunnel: [w735 w737] -> w730
          frame Default {
          }
          frame "Running" {
            n429 = call "MessageQueue_EnqueueElement.vi"("QueueIn"=w741, "Message"="OnlineChangeUM", "ErrorIn"=w738) -> ("QueueOut"=w740:refnum<queue>, "ErrorOut"=w737:errorcluster)  [unwired: 15 in]
          }
        }
      }
      event "Verdichter 1 Gesamtmodell": Value Change {
        n430 = event-data() -> ()  [unwired: 1 in, 6 out]
        n431 = local read "SimState"() -> (w742:T4)
        n432 = case shown="\"Running\"" w742 {
          tunnel: w747 -> [w749 w754]
          tunnel: [w749 w753] -> w746
          tunnel: w744 -> [w748 w751]
          tunnel: [w748 w750] -> w743
          frame Default {
          }
          frame "Running" {
            n433 = call "MessageQueue_EnqueueElement.vi"("QueueIn"=w754, "Message"="OnlineChangeGM", "ErrorIn"=w751) -> ("QueueOut"=w753:refnum<queue>, "ErrorOut"=w750:errorcluster)  [unwired: 15 in]
          }
        }
      }
      event "Verdichter 2 Gesamtmodell": Value Change {
        n434 = event-data() -> ()  [unwired: 1 in, 6 out]
        n435 = local read "SimState"() -> (w755:T4)
        n436 = case shown="\"Running\"" w755 {
          tunnel: w760 -> [w762 w767]
          tunnel: [w762 w766] -> w759
          tunnel: w757 -> [w761 w764]
          tunnel: [w761 w763] -> w756
          frame Default {
          }
          frame "Running" {
            n437 = call "MessageQueue_EnqueueElement.vi"("QueueIn"=w767, "Message"="OnlineChangeGM", "ErrorIn"=w764) -> ("QueueOut"=w766:refnum<queue>, "ErrorOut"=w763:errorcluster)  [unwired: 15 in]
          }
        }
      }
    }
    n438 = Unbundle By Name(w597) -> ("status"=w595:bool)
    n439 = Or(x=w595, y=w598) -> (x .or. y?=w596:bool)
  }
  n440 = Merge Errors(w8, w9) -> (w7:errorcluster)
  n441 = call "MessageQueue_ReleaseQueue.vi"("QueueIn"=w20, "ErrorIn"=w7) -> ("ErrorOut"=w2:errorcluster)  [unwired: 15 in, 2 out]
  n442 = call "ErrorHandling.generalErrorHanlderInclObjRef.vi"("error in"=w2, "Comment(optional)"="SimMainClose" ("Comment")) -> ()  [unwired: 7 in, 3 out]
  n443 = node-c288(w5) -> ()  [unwired: 1 out]
